vi "Preference_Panel.vi"(0 "Mode":T3) -> ()   [LabVIEW 2015]
uses:
  Anemometry Sub Vis/Controls/Server_Comms.ctl
  Anemometry Sub Vis/Controls/Preference_Mode.ctl
  Anemometry Sub Vis/Controls/EnFlo_Data_Folder_Setup.ctl
  Camera Server/sub vis/List of Cameras.ctl
  Anemometry Sub Vis/File/Setup_Filetype.ctl
  Anemometry Sub Vis/Controls/Overhead.ctl
  ADAM Client/Sub VIs/ADAM Controls/Ch_description_ADAM.ctl
  ADAM Client/Sub VIs/ADAM Controls/Module_type_ADAM.ctl
  ADAM Client/Sub VIs/ADAM Controls/Function_ADAM.ctl
  ADAM Client/Sub VIs/ADAM Controls/Channel_State.ctl
  ADAM Client/Sub VIs/ADAM Controls/Calib_type_ADAM.ctl
  ADAM Client/Sub VIs/ADAM Controls/Address.ctl
  Anemometry Sub Vis/Globals/Constants_global.vi
  Anemometry Sub Vis/Globals/Preference_global.vi
  Anemometry Sub Vis/Globals/Trav_pos_global.vi
  Camera Server/Globals/CamServer global.vi
  Anemometry Sub Vis/Acquisition/PWA/PWAtasksGLOBAL.vi
panel:
  in  "Cameras to Log":T1[](array[typedef])
  out "Preferences for computer":string
  in  "Log Cameras if available":bool
  in  "Use New Collision Code":bool
  in  "Traverse to Traverse Collision Detection":bool
  in  "DataTranslation Device No.":u32=20
  in  "Reset Email Counter":bool
  in  "EnFlo_Data_Folder_Setup":T2="EnFlo_Data on Server"
  in  "Post Processing Machine":bool
  in  "Analogue Device Serial No.":string="1188AB4"
  in  "PWA Device Serial No.":string="1187C98"
  in  "ADAM Setup File":u16(ring) items=["Scani_Valve.xls", "Current_Setup.xls"]
  in  "Default Source Establishment Time (s)":dbl=20.0
  out "This Machine's IP Number":string
  in  "Rig Setup":u16(ring) items=["3_x_2_tunnel", "A_Tunnel", "Adam_Sayer_Desk", "ADAM_Server", "Aero_Tunnel", "Alex_Desktop", "B_Tunnel", "Calibration_Tunnel", "Contact_Conductance", "D_Tunnel", "EnFlo_Tunnel", "Frauke_Desktop", "Fruit_Rig", "iMac_G5_2", "iMacDuo1", "Matteo's_desktop", "Matteo_PC", "Nick_PC-2", "Paul_Desk-Paul_Desk_Machine", "Paul_Hayden-Desk", "Paul_N_Desk_Machine_2", "phtest", "Post_Processing_Machine", "PowerBook_G4_1", "PowerBook_G4_2", "Syn_jet_rig", "Tank", "tdf", "Tom_Desk", "Towing_tank", "--New Rig Setup--"]
  in  "Default Traverse Name":u16(ring) items=["A_Tunnel", "Aero_Laser", "Aero_ThroughWall", "Aero_Tunnel", "Angle_Calibrator", "B_Tunnel", "D_Tunnel", "Dummy_Traverse", "EnFlo_Stack", "EnFlo_Tunnel", "EnFlo_Turntable", "Laser_Meas_Traverse", "mohd_setup", "Paul_Desk_Test", "PIV_Traverse", "--New Traverse Setup--"]
  in  "OK":bool
  in  "% Error From First Calib":dbl=10.0 format="%.1f"
  in  "% Error From Previous Calib":dbl=0.5 format="%.1f"
  out "Templates":path=path "/G4_2_HD/Applications (Mac OS 9)/EnFlo Software/Anemometry/Anemometry Sub Vis/Templates"
  in  "Data Folder":path
  out "EnFlo SW Preferences":path=path "/G4_2_HD/Applications (Mac OS 9)/LabVIEW 5.1/EnFlo SW Preferences"
  in  "Tunnel Speed Control":bool
  in  "SMTP server IP address":string
  in  "Abs Press (mbar)":string="Froude:NPL:Atmos_Press"
  in  "Temperature":string="EnFlo Tun:Inlet Heater:Av Temp"
  in  "Server port number":u32=3363
  in  "Server address":string
  in  "LabVIEW Administrators":string[](array[string])=["", "", "", "", "", "", "", "", "", "", "", "", "", "", "", "", "", "", "", ""]
  in  "Server Comms":T4=enum."Do Not Link To Server"
  # "Server Computer Peferences"
  # "Multi Run Preferences"
  # "Warning Levels for Autocalibration Changes"
  # "Email Peferences"
  # "Deg C"
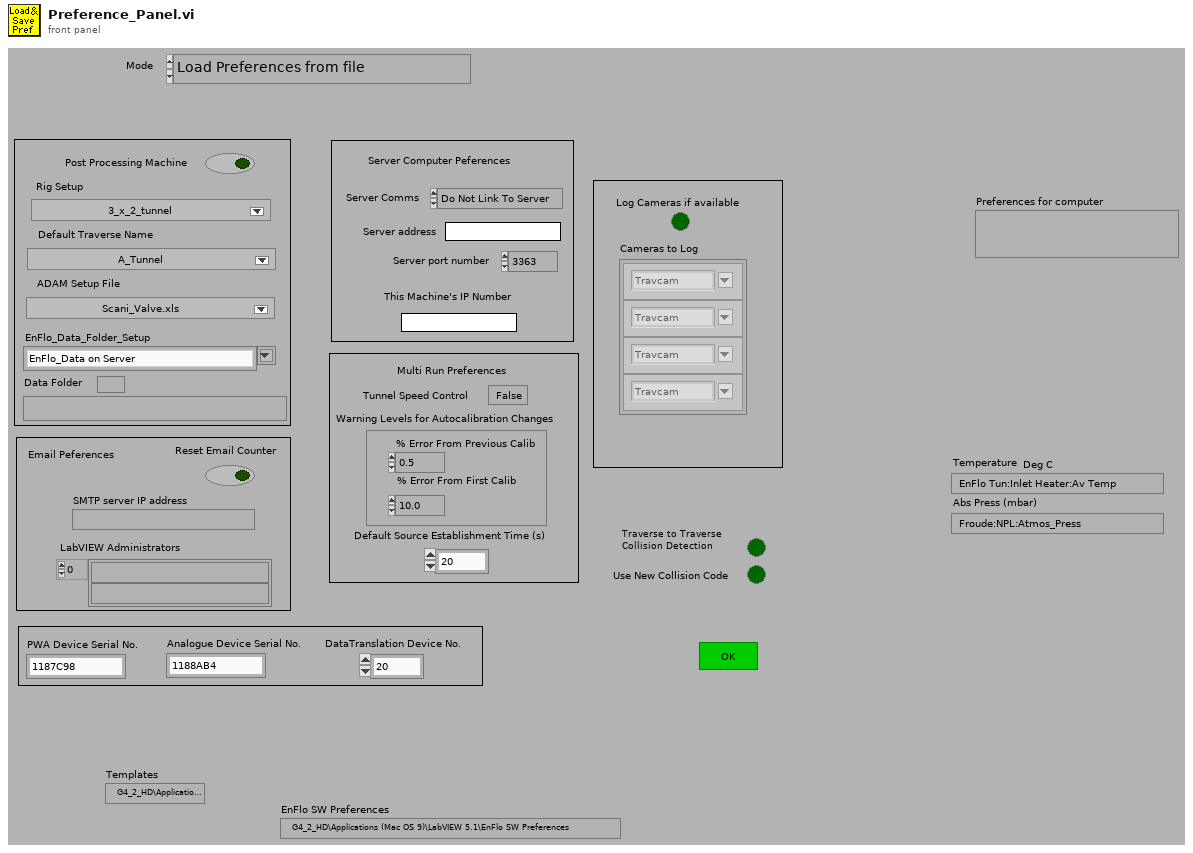
[diagram p1: front panel]
types:
  T1 = typedef "List of Cameras.ctl" = string
  T2 = typedef "EnFlo_Data_Folder_Setup.ctl" = string
  T3 = typedef "Preference_Mode.ctl" = enum16{"Load Preferences from file", "Save Preferences to file", "Load, Edit then Save"}
  T4 = typedef "Server_Comms.ctl" = enum16{"Server Link Healthy", "Do Not Link To Server"}
  T5 = enum16{"Zero or one", "One", "Zero or more", "One or more"}
  T6 = enum8{"Enabled", "Disabled", "Disabled and Grayed Out"}
  T7 = typedef "Setup_Filetype.ctl" = enum16{"Measurement Setups", "Calibration Setups", "General", "Results File Plotter Setups", "Speed Calib Tweaks"}
  T8 = typedef "Overhead.ctl" = enum16{"Update total times", "Read Current Overhead", "Re Scale totals to 3 hrs", "Initialise totals to 3hr"}
  T9 = typedef "Calib_type_ADAM.ctl" = enum16{"Raw", "Bx + A", "Cx^2 + Bx + A", "Dx^3 + Cx^2 + Bx + A", "In Band", "Hi-Tec Q", "Hi-Tec M_dot", "Text"}
  T10 = typedef "Module_type_ADAM.ctl" = string
  T11 = typedef "Channel_State.ctl" = enum16{"On", "Off", "Always On", "Always Off"}
  T12 = typedef "LVDateTimeRec.ctl" = cluster{"fractional second":dbl, "second":i32, "minute":i32, "hour":i32, "day of month":i32, "month":i32, "year":i32, "day of week":i32, "day of year":i32, "DST":i32}
  T13 = typedef "Ch_description_ADAM.ctl" = cluster{"Ch Name":string, "Type":T10, "Function":T14, "Ch State":T11, "Calibration type":T9, "A":dbl, "B":dbl, "C":dbl, "D":dbl, "Comments":string, "Address":T15, "String":string, "Duty":u16}
  T14 = typedef "Function_ADAM.ctl" = enum16{"Analogue Input", "Digital Input", "Event counter", "Event rate", "Analogue Output", "Digital Output", "Relay Output"}
  T15 = typedef "Address.ctl" = cluster{"Main":i32, "Ch.":i32, "Sub":i32, "Port Name":string}
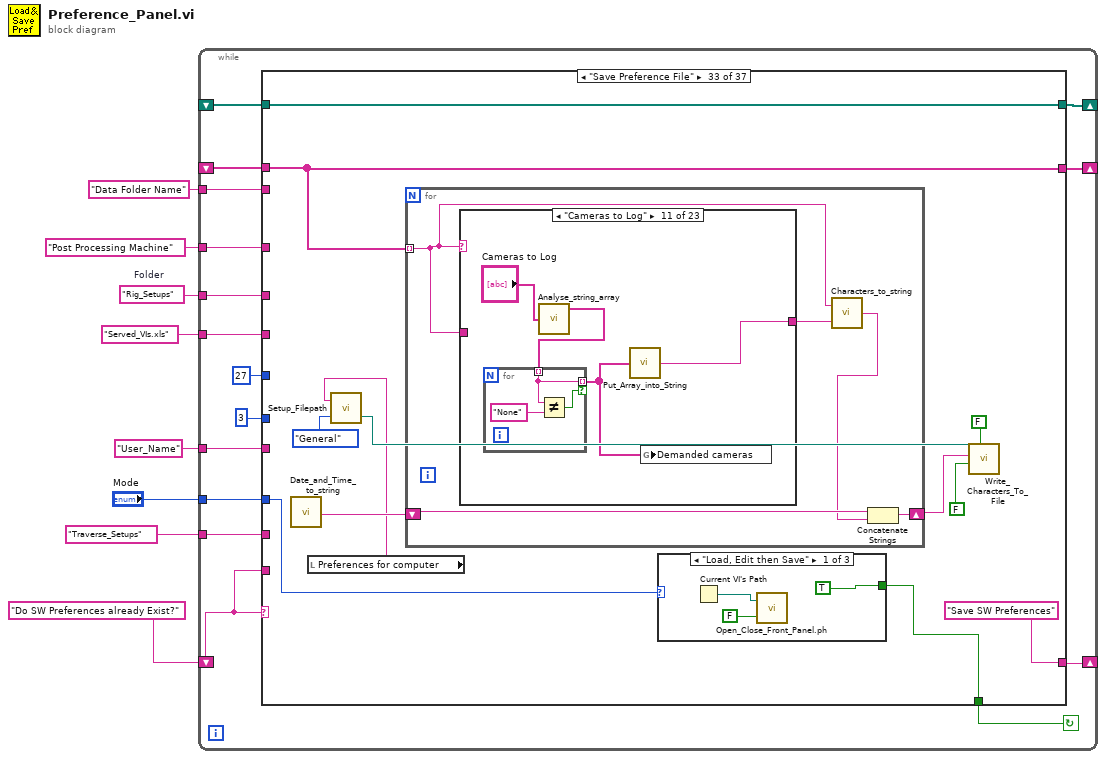
[diagram p0: block diagram]
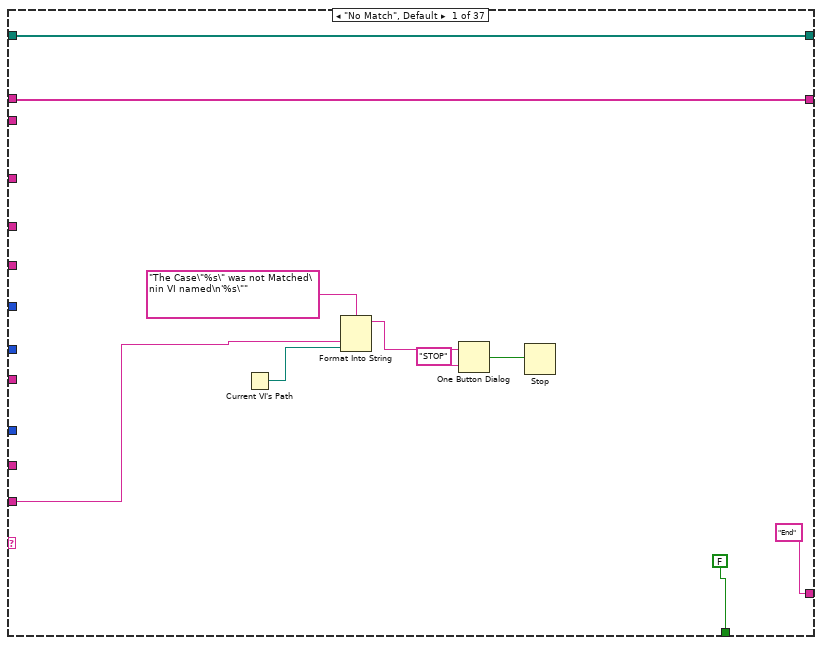
[diagram p2: hidden frame]
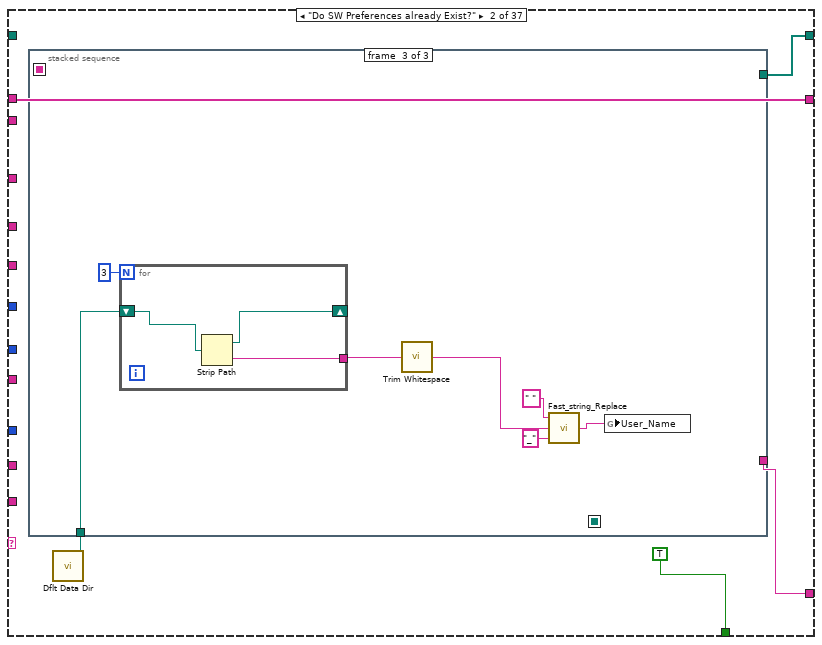
[diagram p3: hidden frame]
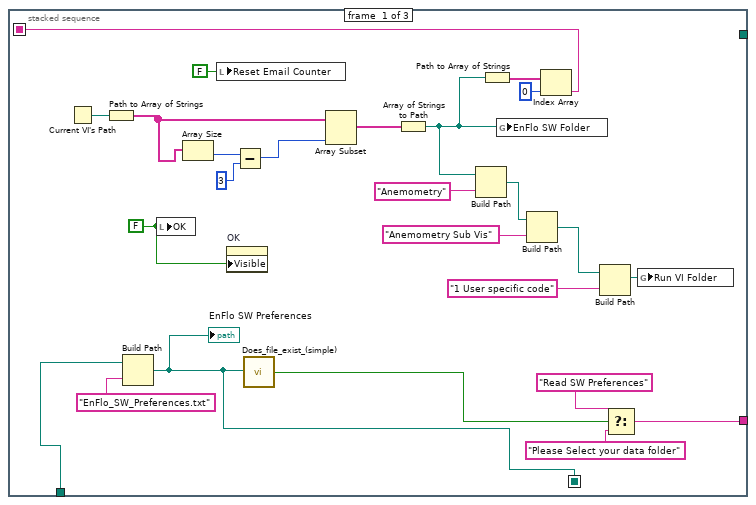
[diagram p4: hidden frame]
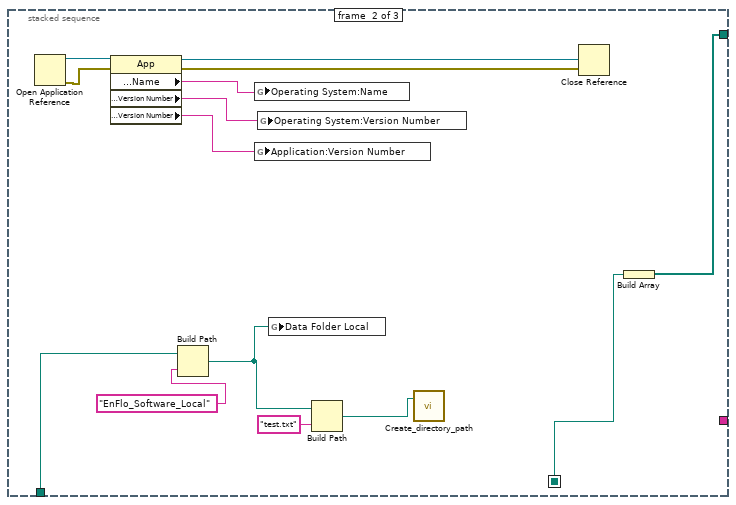
[diagram p5: hidden frame]
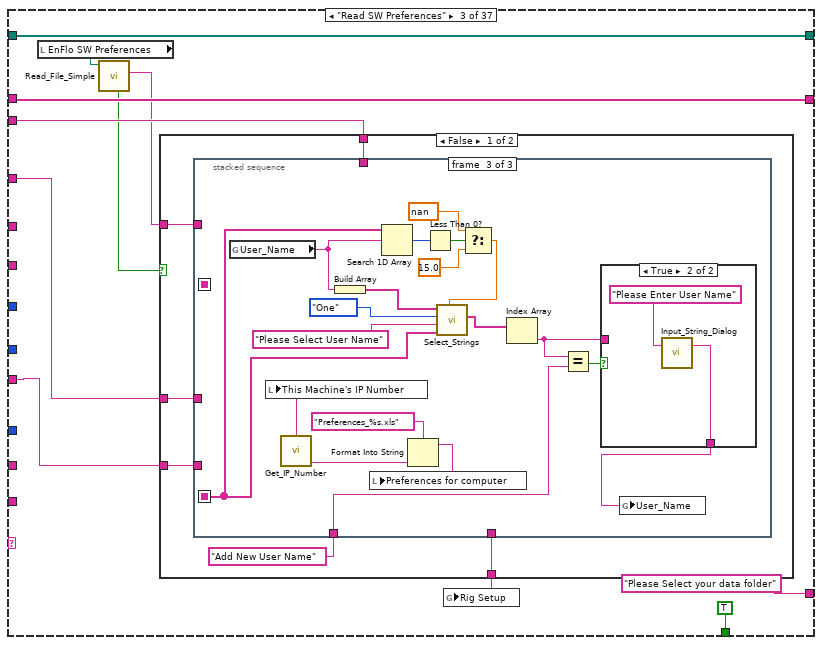
[diagram p6: hidden frame]
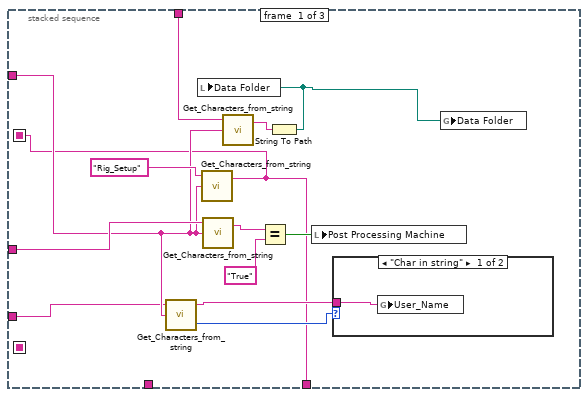
[diagram p7: hidden frame]
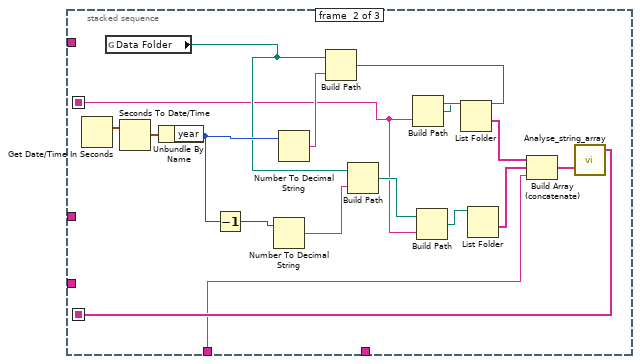
[diagram p9: hidden frame]
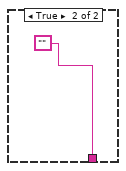
[diagram p11: hidden frame]
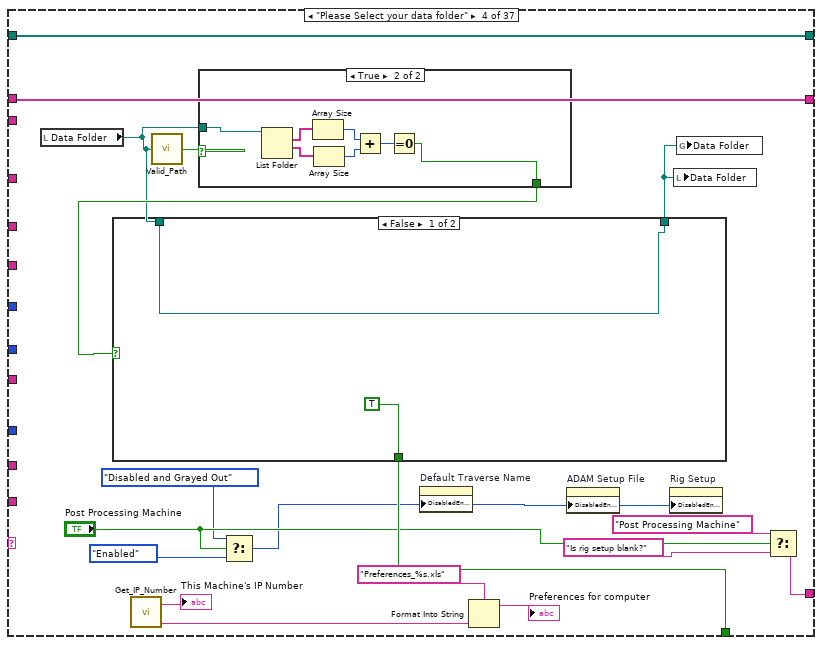
[diagram p12: hidden frame]
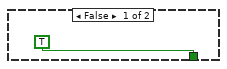
[diagram p13: hidden frame]
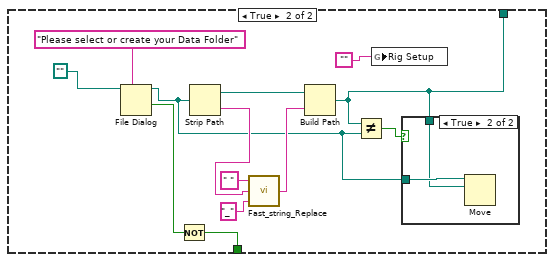
[diagram p14: hidden frame]
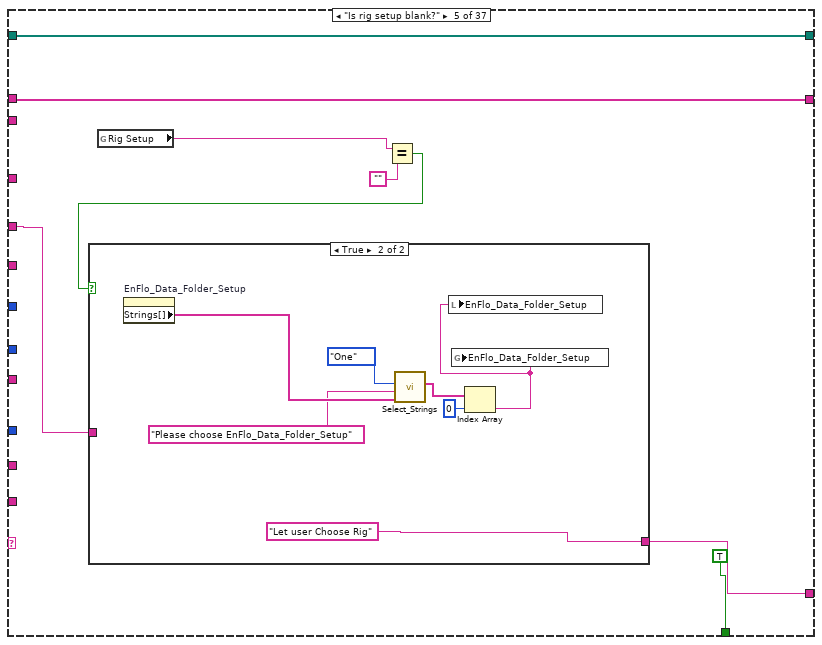
[diagram p16: hidden frame]
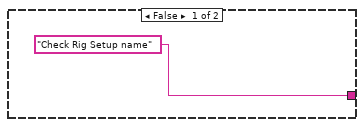
[diagram p17: hidden frame]
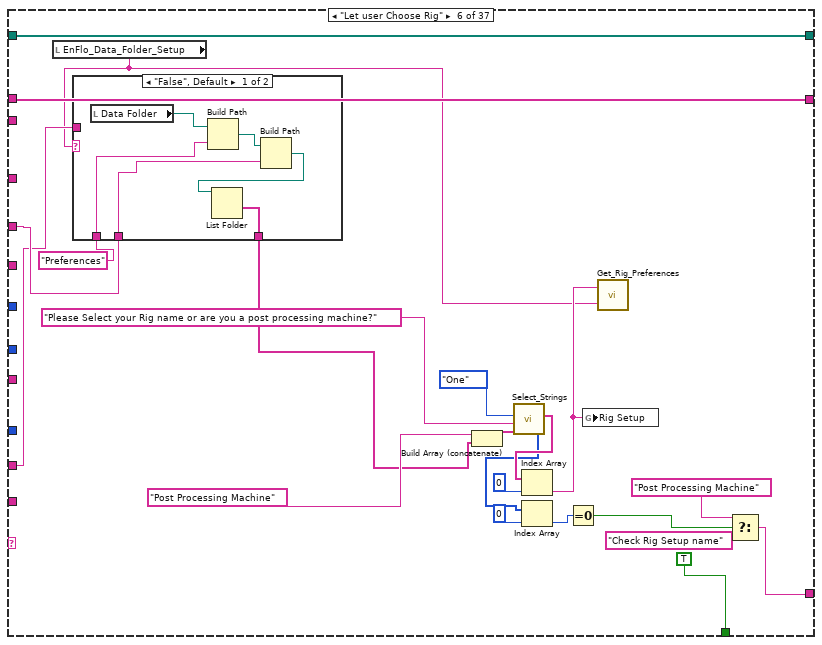
[diagram p18: hidden frame]
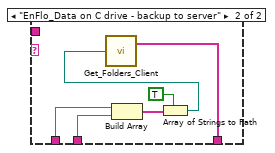
[diagram p19: hidden frame]
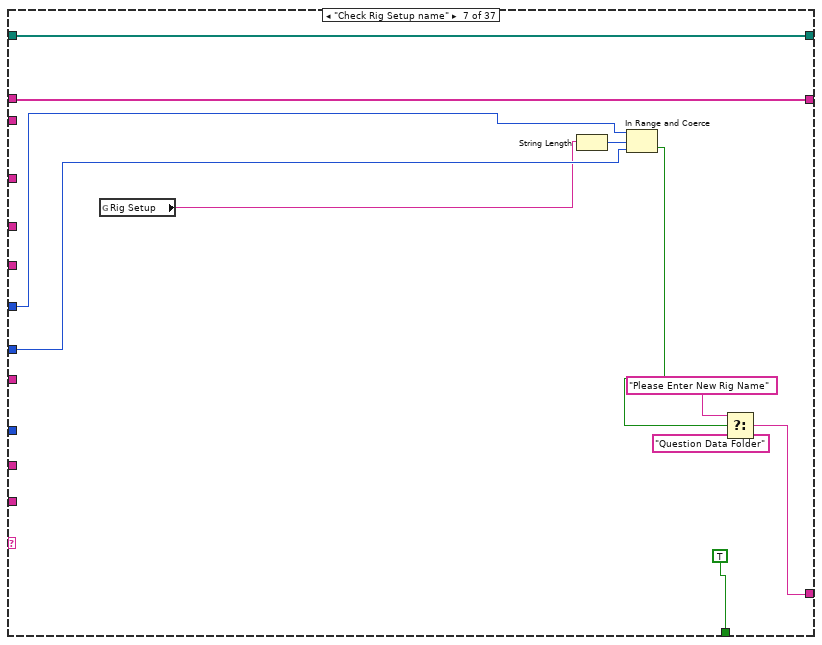
[diagram p20: hidden frame]
diagram:
  w4 = "Rig_Setups"  # Folder
  n1 = while {
    shift-left: _ -> [w21]
    shift-right: [w22] -> _
    shift-left: "Do SW Preferences already Exist?" -> [w10]
    shift-right: [w23] -> _
    tunnel: "Mode" -> [w20]
    tunnel: "Data Folder Name" ("Label for characters") -> [w19]
    tunnel: "Served_VIs.xls" ("Substring") -> [w18]
    tunnel: w4 -> [w15]
    tunnel: "Traverse_Setups" ("name or relative path") -> [w14]
    shift-right: [w13] -> _
    shift-left: _ -> [w12]
    tunnel: "Post Processing Machine" ("Label for characters") -> [w11]
    tunnel: "User_Name" ("Label for characters") -> [w9]
    stop <- w24 continue-if-true
    n2 = case shown="\"Save Preference File\"" w10 {
      tunnel: [FALSE TRUE TRUE w171 TRUE TRUE TRUE TRUE TRUE TRUE TRUE TRUE TRUE TRUE TRUE TRUE TRUE TRUE TRUE TRUE TRUE TRUE TRUE TRUE TRUE TRUE TRUE TRUE TRUE TRUE TRUE TRUE w938 TRUE TRUE TRUE FALSE] -> w24
      tunnel: ["End" w37 "Please Select your data folder" w168 w203 w236 w253 w264 w283 "Update Constants Global" ("f") "Copy Preferences?" "Copy Preferences?" w414 w431 "Install Preference files" "Install Adam table files" "Install Adam setup files" "Choose ADAM Setup file" "Preference files continued" "Variable Names" w611 w631 "Please Enter new  Traverse Setup" w718 "Create Traverse setup" ("f") "Check file permission status" w815 w846 w866 w886 w902 "Save Preference File" "Save SW Preferences" w1028 w1042 "Initialise Globals" "End"] -> w23
      tunnel: [w26 w38 w98 w177 w209 w239 w262 w272 w285 w350 w378 w401 w412 w435 w493 w508 w533 w552 w574 w584 w616 w638 w706 w720 w754 w771 w816 w851 w871 w894 w907 w927 w944 w1036 w1043 w1095 w1153] -> w22
      tunnel: w21 -> [w26 w38 w98 w177 w209 w239 w262 w272 w285 w350 w378 w401 w412 w435 w493 w508 w533 w552 w574 w584 _ w638 w706 w720 w754 w771 w816 w851 w871 w894 w907 w927 w944 w1036 w1043 w1095 w1153]
      tunnel: w10 -> [w29 _ _ _ _ _ _ _ _ _ _ _ _ _ _ _ _ _ _ _ _ _ _ _ _ _ _ _ _ _ _ _ _ _ _ _ _]
      tunnel: w20 -> [_ _ _ _ _ _ _ _ _ _ _ _ _ _ _ _ _ _ _ _ w610 _ _ _ _ _ w814 _ _ _ _ _ w939 _ _ _ _]
      tunnel: w19 -> [_ _ w95 _ _ _ _ _ _ _ _ _ _ _ _ _ _ _ _ _ _ _ _ _ _ _ _ _ _ _ _ _ _ w1027 _ _ _]
      tunnel: w18 -> [_ _ _ _ _ _ _ _ _ _ _ _ _ _ _ w503 _ _ _ _ _ _ _ _ _ _ _ _ _ _ _ _ _ _ _ w1087 _]
      tunnel: 3 ("lower limit") -> [_ _ _ _ _ _ w258 _ w282 _ _ _ _ _ _ _ _ _ _ _ _ _ _ w717 _ _ _ _ _ _ _ _ _ _ _ _ _]
      tunnel: 27 ("upper limit") -> [_ _ _ _ _ _ w259 _ w281 _ _ _ _ _ _ _ _ _ _ _ _ _ _ w716 _ _ _ _ _ _ _ _ _ _ _ _ _]
      tunnel: w15 -> [_ _ _ _ w206 w224 _ _ _ w338 w366 _ _ w434 _ _ _ _ _ _ _ _ _ _ _ _ _ _ _ _ _ _ _ _ _ _ _]
      tunnel: w14 -> [_ _ _ _ _ w221 _ _ _ _ _ _ _ _ _ _ _ _ _ _ _ _ w704 _ w741 _ _ _ _ _ _ _ _ _ _ _ _]
      tunnel: [w25 w35 w94 w172 w204 w238 w261 w271 w277 w336 w363 w390 w413 w436 w486 w500 w526 w549 w560 w576 w603 w634 w703 w712 w740 w767 path[] [] w843 w863 w889 w905 w926 w937 w1024 w1041 w1089 w1151] -> w13
      tunnel: w12 -> [w25 _ w94 w172 w204 w238 w261 w271 w277 w336 w363 w390 w413 w436 w485 w502 w526 w550 w560 w578 w603 w635 w703 w712 w740 w768 w813 w843 w863 w889 w905 w926 w937 w1024 w1041 w1089 w1151]
      tunnel: w11 -> [_ _ w93 _ _ _ _ _ _ _ _ _ _ _ _ _ _ _ _ _ _ _ _ _ _ _ _ _ _ _ _ _ _ w1018 _ _ _]
      tunnel: w9 -> [_ _ w89 _ _ _ _ _ _ _ _ _ _ _ _ _ _ _ _ _ _ _ _ _ _ _ _ _ _ _ _ _ _ w1017 _ _ _]
      frame "No Match", Default {
        n3 = Current VI's Path() -> (path=w34:path)
        n4 = Format Into String(format string="The Case\"%s\" was not Matched\nin VI named\n'%s\"" ("Format String"), w29, w34) -> (resulting string=w31:string)  [unwired: 2 in, 1 out]
        n5 = One Button Dialog(message=w31, button name ("OK")="STOP") -> (true=w33:bool)
        n6 = Stop(stop? (T)=w33) -> ()
      }
      frame "Do SW Preferences already Exist?" {
        n7 = call <vilib>:"Dflt Data Dir.vi"() -> ("App:Default Data Directory"=w36:path)
        n8 = stacked-sequence {
          seq-local: [w44 _ _] -> [_ _ _]
          seq-local: [w42 _ _] -> [_ w70 _]
          tunnel: [w48 _ _] -> w37
          tunnel: w36 -> [w43 w68 w84]
          tunnel: [_ w71 _] -> w35
          frame #0 {
            w41 = FALSE ("OK")
            n9 = Current VI's Path() -> (path=w62:path)
            n10 = Path to Array of Strings(0:w62) -> (2:w59:string[])  [unwired: 1 out]
            n11 = Build Path(base path=w43, name or relative path="EnFlo_SW_Preferences.txt") -> (appended path=w42:path)
            "EnFlo SW Preferences" <- w42
            n12 = local write "OK"(w41) -> ()
            n13 = Array Size(array=w59) -> (size(s)=w61:i32)
            n14 = local write "Reset Email Counter"(FALSE ("Reset Email Counter")) -> ()
            n15 = property on="OK" class="Bool (strict)"("Visible"=w41) -> ()  [unwired: 2 in, 2 out]
            n16 = Subtract(x=w61, y=3) -> (x-y=w57:i32)
            n17 = call "Does_file_exist_(simple).vi"("Pathname"=w42) -> ("exists?"=w63:bool)
            n18 = Array Subset(array=w59, length=w57) -> (w58:string[])  [unwired: 1 in]
            n19 = Array of Strings to Path(0:w58) -> (2:w45:path)  [unwired: 1 out]
            n20 = Build Path(base path=w45, name or relative path="Anemometry") -> (appended path=w54:path)
            n21 = Path to Array of Strings(0:w45) -> (2:w46:string[])  [unwired: 1 out]
            n22 = global write "Constants_global.vi" "EnFlo SW Folder"(w45) -> ()
            n23 = Build Path(base path=w54, name or relative path="Anemometry Sub Vis") -> (appended path=w52:path)
            n24 = Index Array(array=w46, index=0) -> (element=w44:string)
            n25 = Build Path(base path=w52, name or relative path="1 User specific code") -> (appended path=w51:path)
            n26 = Select(t="Read SW Preferences", s=w63, f="Please Select your data folder") -> (s? t:f=w48:string)
            n27 = global write "Constants_global.vi" "Run VI Folder"(w51) -> ()
          }
          frame #1 {
            n28 = Open Application Reference() -> (0:w75:errorcluster, 3:w78:refnum<vi>)  [unwired: 1 in, 3 out]
            n29 = property class="App"(reference=w78, error in=w75) -> (reference out=w77:refnum<vi>, error out=w76:errorcluster, "Operating System:Name"=w72:string, "Operating System:Version Number"=w74:string, "Application:Version Number"=w73:string)
            n30 = Build Path(base path=w68, name or relative path="EnFlo_Software_Local" ("element")) -> (appended path=w67:path)
            n31 = global write "Preference_global.vi" "Operating System:Name"(w72) -> ()
            n32 = global write "Preference_global.vi" "Application:Version Number"(w73) -> ()
            n33 = global write "Preference_global.vi" "Operating System:Version Number"(w74) -> ()
            n34 = global write "Constants_global.vi" "Data Folder Local"(w67) -> ()
            n35 = Build Path(base path=w67, name or relative path="test.txt") -> (appended path=w65:path)
            n36 = call "Create_directory_path.vi"("Path name"=w65) -> ()  [unwired: 1 in, 2 out]
            n37 = Close Reference(reference=w77, error in (no error)=w76) -> ()  [unwired: 1 out]
            n38 = Build Array(w70) -> (w71:path[])
          }
          frame #2 {
            n39 = for {
              N: 3 -> [_]
              shift-right: [w88] -> _
              shift-left: w84 -> [w87]
              tunnel: [w86] -> w80
              n40 = Strip Path(path=w87) -> (stripped path=w88:path, name=w86:string)
            }
            n41 = call <vilib>:"Trim Whitespace.vi"("string"=w80) -> ("trimmed string"=w79:string)  [unwired: 1 in]
            n42 = call "Fast_string_Replace.vi"("Replace match with:"="_", "Input String"=w79, "regular expression"=" ") -> ("Output String"=w81:string)  [unwired: 1 in, 1 out]
            n43 = global write "Preference_global.vi" "User_Name"(w81) -> ()
          }
        }
      }
      frame "Read SW Preferences" {
        n44 = local read "EnFlo SW Preferences"() -> (w97:path)
        n45 = call "Read_File_Simple.vi"("Filename"=w97) -> ("Error?"=w91:bool, "string"=w92:string)  [unwired: 2 in, 6 out]
        n46 = case shown="False" w91 {
          tunnel: w95 -> [w105 _]
          tunnel: w93 -> [w104 _]
          tunnel: w92 -> [w102 _]
          tunnel: [w103 ""] -> w90
          tunnel: w89 -> [w101 _]
          frame False {
            n47 = stacked-sequence {
              seq-local: [w106 _ _] -> [_ w126 _]
              seq-local: [_ w121 _] -> [_ _ w146]
              tunnel: w105 -> [w117 _ _]
              tunnel: w104 -> [w114 _ _]
              tunnel: [w106 _ _] -> w103
              tunnel: w102 -> [w110 _ _]
              tunnel: w101 -> [w109 _ _]
              tunnel: "Add New User Name" -> [_ w120 w151]
              frame #0 {
                n48 = call "Get_Characters_from_string.vi"("Input string"=w110, "Variable name"=w109) -> ("Status"=w108:enum16{"Char in string", "Char not in string"}, "Value"=w107:string)  [unwired: 1 in]
                n49 = call "Get_Characters_from_string.vi"("Input string"=w110, "Variable name"="Rig_Setup" ("Label for characters")) -> ("Value"=w106:string)  [unwired: 1 in, 1 out]
                n50 = call "Get_Characters_from_string.vi"("Input string"=w110, "Variable name"=w114) -> ("Value"=w113:string)  [unwired: 1 in, 1 out]
                n51 = call "Get_Characters_from_string.vi"("Input string"=w110, "Variable name"=w117) -> ("Value"=w118:string)  [unwired: 1 in, 1 out]
                n52 = Equal?(x=w113, y="True") -> (x = y?=w111:bool)
                n53 = String To Path(string=w118) -> (path=w116:path)
                n54 = local write "Data Folder"(w116) -> ()
                n55 = local write "Post Processing Machine"(w111) -> ()
                n56 = case shown="\"Char in string\"" w108 {
                  tunnel: w107 -> [w119 _]
                  frame "Char in string" {
                    n57 = global write "Preference_global.vi" "User_Name"(w119) -> ()
                  }
                  frame "Char not in string" {
                  }
                }
                n58 = global write "Constants_global.vi" "Data Folder"(w116) -> ()
              }
              frame #1 {
                n59 = Get Date/Time In Seconds() -> (seconds since 1Jan1904=w136:timestamp)
                n60 = global read "Constants_global.vi" "Data Folder"() -> (w129:path)
                n61 = Seconds To Date/Time(time stamp (now)=w136) -> (date time rec=w135:T12)  [unwired: 1 in]
                n62 = Unbundle By Name(w135) -> ("year"=w134:i32)
                n63 = Decrement(x=w134) -> (x-1=w133:i32)
                n64 = Number To Decimal String(number=w133) -> (decimal integer string=w128:string)  [unwired: 1 in]
                n65 = Number To Decimal String(number=w134) -> (decimal integer string=w132:string)  [unwired: 1 in]
                n66 = Build Path(base path=w129, name or relative path=w132) -> (appended path=w131:path)
                n67 = Build Path(base path=w129, name or relative path=w128) -> (appended path=w127:path)
                n68 = Build Path(base path=w131, name or relative path=w126) -> (appended path=w130:path)
                n69 = Build Path(base path=w127, name or relative path=w126) -> (appended path=w125:path)
                n70 = List Folder(path=w130) -> (folder names=w124:string[])  [unwired: 3 in, 3 out]
                n71 = List Folder(path=w125) -> (folder names=w123:string[])  [unwired: 3 in, 3 out]
                n72 = Build Array (concatenate)(w124, w123, w120) -> (w122:string[])
                n73 = call "Analyse_string_array.vi"("String array"=w122) -> ("Unique strings"=w121:string[])  [unwired: 1 in, 1 out]
              }
              frame #2 {
                n74 = global read "Preference_global.vi" "User_Name"() -> (w147:string)
                n75 = call "Get_IP_Number.vi"() -> ("Computer Name"=w139:string, "IP Number"=w140:string)
                n76 = local write "This Machine's IP Number"(w140) -> ()
                n77 = Build Array(w147) -> (w154:string[])
                n78 = Search 1D Array(1D array=w146, element=w147) -> (index of element=w145:i32)  [unwired: 1 in]
                n79 = Format Into String(format string="Preferences_%s.xls" ("name or relative path"), w139) -> (resulting string=w138:string)  [unwired: 2 in, 1 out]
                n80 = local write "Preferences for computer"(w138) -> ()
                n81 = Less Than 0?(x=w145) -> (x < 0?=w144:bool)
                n82 = Select(t=nan ("Timeout (s)"), s=w144, f=15.0 ("Timeout (s)")) -> (s? t:f=w141:dbl)
                n83 = call "Select_Strings.vi"("Timeout (s)"=w141, "Available Ch names"=w146, "Message"="Please Select User Name", "Selector mode"=T5."One", "Desired Ch names (in)"=w154) -> ("Selected Channel Names"=w152:string[])  [unwired: 1 in, 2 out]
                n84 = Index Array(array=w152) -> (element=w148:string)  [unwired: 1 in]
                n85 = Equal?(x=w148, y=w151) -> (x = y?=w150:bool)
                n86 = case shown="True" w150 {
                  tunnel: [w156 w157] -> w149
                  tunnel: w148 -> [w156 _]
                  frame False {
                  }
                  frame True {
                    n87 = call "Input_String_Dialog.vi"("Message to user"="Please Enter User Name") -> ("Output string"=w157:string)  [unwired: 1 in, 1 out]
                  }
                }
                n88 = global write "Preference_global.vi" "User_Name"(w149) -> ()
              }
            }
          }
          frame True {
          }
        }
        n89 = global write "Preference_global.vi" "Rig Setup"(w90) -> ()
      }
      frame "Please Select your data folder" {
        n90 = local read "Data Folder"() -> (w173:path)
        n91 = call "Get_IP_Number.vi"() -> ("Computer Name"=w162:string, "IP Number"=→"This Machine's IP Number":string)
        n92 = call "Valid_Path.vi"("Filename"=w173) -> ("Valid Path?"=w175:bool)
        n93 = case shown="True" w175 {
          tunnel: [TRUE ("status") w179] -> w174
          tunnel: w173 -> [_ w185]
          frame False {
          }
          frame True {
            n94 = List Folder(path=w185) -> (filenames=w183:string[], folder names=w184:string[])  [unwired: 1 in, 4 out]
            n95 = Array Size(array=w183) -> (size(s)=w181:i32)
            n96 = Array Size(array=w184) -> (size(s)=w182:i32)
            n97 = Add(x=w181, y=w182) -> (x+y=w180:i32)
            n98 = Equal To 0?(x=w180) -> (x = 0?=w179:bool)
          }
        }
        n99 = case shown="False" w174 {
          tunnel: [w187 w191] -> w176
          tunnel: w173 -> [w187 _]
          tunnel: [TRUE w189] -> w171
          frame False {
          }
          frame True {
            n100 = File Dialog(7:"Please select or create your Data Folder" ("prompt"), 11:path "") -> (1:w190:bool, 3:w192:path)  [unwired: 1 in, 6 out]
            n101 = Not(x=w190) -> (.not. x?=w189:bool)
            n102 = Strip Path(path=w192) -> (stripped path=w196:path, name=w195:string)
            n103 = call "Fast_string_Replace.vi"("Replace match with:"="_", "Input String"=w195, "regular expression"=" ") -> ("Output String"=w194:string)  [unwired: 2 out]
            n104 = Build Path(base path=w196, name or relative path=w194) -> (appended path=w191:path)
            n105 = Not Equal?(x=w191, y=w192) -> (x != y?=w193:bool)
            n106 = global write "Preference_global.vi" "Rig Setup"("") -> ()
            n107 = case shown="True" w193 {
              tunnel: w192 -> [_ w202]
              tunnel: w191 -> [_ w201]
              frame False {
              }
              frame True {
                n108 = Move(source path=w202, 10:w201) -> ()  [unwired: 1 in, 5 out]
              }
            }
          }
        }
        n109 = Select(t=T6."Disabled and Grayed Out" ("Disabled"), s="Post Processing Machine", f=T6."Enabled" ("Disabled")) -> (s? t:f=w164:T6)
        n110 = property on="Default Traverse Name" class="Ring (strict)"("DisabledEnum"=w164) -> ()  [unwired: 2 in, 2 out]
        n111 = Format Into String(format string="Preferences_%s.xls" ("name or relative path"), w162) -> (resulting string=→"Preferences for computer":string)  [unwired: 2 in, 1 out]
        n112 = property on="ADAM Setup File" class="Ring (strict)"("DisabledEnum"=w164) -> ()  [unwired: 2 in, 2 out]
        n113 = property on="Rig Setup" class="Ring (strict)"("DisabledEnum"=w164) -> ()  [unwired: 2 in, 2 out]
        n114 = local write "Data Folder"(w176) -> ()
        n115 = global write "Constants_global.vi" "Data Folder"(w176) -> ()
        n116 = Select(t="Post Processing Machine", s="Post Processing Machine", f="Is rig setup blank?") -> (s? t:f=w168:string)
      }
      frame "Is rig setup blank?" {
        n117 = global read "Preference_global.vi" "Rig Setup"() -> (w205:string)
        n118 = Equal?(x=w205, y="") -> (x = y?=w207:bool)
        n119 = case shown="True" w207 {
          tunnel: w206 -> [_ _]
          tunnel: ["Check Rig Setup name" ("t") "Let user Choose Rig"] -> w203
          frame False {
          }
          frame True {
            n120 = property on="EnFlo_Data_Folder_Setup" class="CmbBox (strict)"() -> ("Strings[]"=w216:string[])  [unwired: 2 in, 2 out]
            n121 = call "Select_Strings.vi"("Available Ch names"=w216, "Message"="Please choose EnFlo_Data_Folder_Setup", "Selector mode"=T5."One") -> ("Selected Channel Names"=w214:string[])  [unwired: 3 in, 2 out]
            n122 = Index Array(array=w214, index=0) -> (element=w212:string)
            n123 = local write "EnFlo_Data_Folder_Setup"(w212) -> ()
            n124 = global write "Preference_global.vi" "EnFlo_Data_Folder_Setup"(w212) -> ()
          }
        }
      }
      frame "Let user Choose Rig" {
        n125 = local read "EnFlo_Data_Folder_Setup"() -> (w219:T2)
        n126 = case shown="\"False\", Default" w219 {
          tunnel: "Preferences" ("name or relative path") -> [w244 w247]
          tunnel: w224 -> [w243 w252]
          tunnel: [w242 w249] -> w222
          tunnel: w221 -> [_ _]
          frame "False", Default {
            n127 = local read "Data Folder"() -> (w245:path)
            n128 = Build Path(base path=w245, name or relative path=w244) -> (appended path=w246:path)
            n129 = Build Path(base path=w246, name or relative path=w243) -> (appended path=w241:path)
            n130 = List Folder(path=w241) -> (folder names=w242:string[])  [unwired: 1 in, 5 out]
          }
          frame "EnFlo_Data on C drive - backup to server" {
            n131 = Build Array(w247, w252) -> (w251:string[])
            n132 = Array of Strings to Path(0:w251, 1:TRUE ("relative")) -> (2:w248:path)
            n133 = call "Get_Folders_Client.vi"("Relative Path"=w248) -> ("Folder Names"=w249:string[])  [unwired: 1 out]
          }
        }
        n134 = Build Array (concatenate)("Post Processing Machine", w222) -> (w229:string[])
        n135 = call "Select_Strings.vi"("Available Ch names"=w229, "Message"="Please Select your Rig name or are you a post processing machine?", "Selector mode"=T5."One") -> ("Ch Indicies Choosen"=w226:i32[], "Selected Channel Names"=w228:string[])  [unwired: 3 in, 1 out]
        n136 = Index Array(array=w228, index=0) -> (element=w220:string)
        n137 = Index Array(array=w226, index=0) -> (element=w225:i32)
        n138 = Equal To 0?(x=w225) -> (x = 0?=w235:bool)
        n139 = global write "Preference_global.vi" "Rig Setup"(w220) -> ()
        n140 = call "Get_Rig_Preferences.vi"("EnFlo_Data_Folder_Setup"=w219, "Rig Setup"=w220) -> ()  [unwired: 1 in]
        n141 = Select(t="Post Processing Machine", s=w235, f="Check Rig Setup name") -> (s? t:f=w236:string)
      }
      frame "Check Rig Setup name" {
        n142 = global read "Preference_global.vi" "Rig Setup"() -> (w254:string)
        n143 = String Length(string=w254) -> (length=w260:i32)
        n144 = In Range and Coerce(upper limit=w259, x=w260, lower limit=w258) -> (In Range?=w257:bool)  [unwired: 1 out]
        n145 = Select(t="Please Enter New Rig Name", s=w257, f="Question Data Folder") -> (s? t:f=w253:string)
      }
      frame "Question Data Folder" {
        (unwired) "Question Data Folder"
        n146 = local read "Data Folder"() -> (w270:path)
        n147 = Format Into String(format string="Is the Data Folder\n%s\nCorrect?" ("message"), w270) -> (resulting string=w268:string)  [unwired: 2 in, 1 out]
        n148 = Two Button Dialog(message=w268, 1:"No, let me change it" ("F button name (\"Cancel\")"), 2:"Yes" ("T button name (\"OK\")")) -> (T button?=w265:bool)
        n149 = case shown="False" w265 {
          tunnel: ["Please Select your data folder" "Please Enter New Rig Name"] -> w264
          frame False {
            n150 = local write "Data Folder"(path "") -> ()
          }
          frame True {
          }
        }
      }
      frame "Please Enter New Rig Name" {
        n151 = global read "Preference_global.vi" "Rig Setup"() -> (w279:string)
        n152 = String Length(string=w279) -> (length=w284:i32)
        n153 = In Range and Coerce(upper limit=w281, x=w284, lower limit=w282) -> (In Range?=w280:bool)  [unwired: 1 out]
        n154 = case shown="False" w280 {
          tunnel: w279 -> [w291 w334]
          tunnel: [w287 "Update Rig setup menu ring"] -> w283
          tunnel: [w288 w334] -> w278
          tunnel: w282 -> [w290 _]
          tunnel: w281 -> [w289 _]
          frame False {
            n155 = stacked-sequence {
              seq-local: [w292 _] -> [_ w317]
              seq-local: [w299 _] -> [_ _]
              tunnel: w291 -> [w301 _]
              tunnel: w290 -> [w312 _]
              tunnel: w289 -> [w298 w315]
              tunnel: [_ w320] -> w288
              tunnel: [w304 _] -> w287
              frame #0 {
                n156 = Match Pattern(string=w301, regular expression="-") -> (before substring=w300:string, after substring=w299:string)  [unwired: 3 out]
                n157 = String Length(string=w299) -> (length=w297:i32)
                n158 = Subtract(x=w298, y=w297) -> (x-y=w296:i32)
                n159 = Format Into String(format string="Please Enter a Rig Name.\n It must be between %d and %d Characters" ("Message to user"), w312, w296) -> (resulting string=w311:string)  [unwired: 2 in, 1 out]
                n160 = call "Input_String_Dialog.vi"("Value"=w300, "Message to user"=w311) -> ("Ok Out"=w307:bool, "Output string"=w308:string)
                n161 = call "Fast_string_Replace.vi"("Replace match with:"="_", "Input String"=w308, "regular expression"=" ") -> ("Output String"=w293:string)  [unwired: 2 out]
                n162 = Select(t="Please Enter New Rig Name", s=w307, f="Save Preference File") -> (s? t:f=w304:string)
                n163 = call "Fast_string_Replace.vi"("Replace match with:"="_", "Input String"=w293, "regular expression"="-") -> ("Output String"=w292:string)  [unwired: 2 out]
              }
              frame #1 {
                n164 = String Length(string=w317) -> (length=w316:i32)
                n165 = Subtract(x=w315, y=w316) -> (x-y=w314:i32)
                n166 = Format Into String(format string="Please Enter a Rig Machine identifier if more than one machine per Rig.\n(Leave Blank for Rigs only using one Machine.)\nMust be less than %d Characters." ("Message to user"), w314) -> (resulting string=w313:string)  [unwired: 2 in, 1 out]
                n167 = call "Input_String_Dialog.vi"("Value"="", "Message to user"=w313) -> ("Output string"=w326:string)  [unwired: 1 out]
                n168 = call "Fast_string_Replace.vi"("Replace match with:"="_", "Input String"=w326, "regular expression"=" ") -> ("Output String"=w322:string)  [unwired: 2 out]
                n169 = call "Fast_string_Replace.vi"("Replace match with:"="_", "Input String"=w322, "regular expression"="-") -> ("Output String"=w319:string)  [unwired: 2 out]
                n170 = Empty String/Path?(string/path=w319) -> (empty?=w321:bool)
                n171 = case shown="False" w321 {
                  tunnel: [w329 w333] -> w320
                  tunnel: w317 -> [w332 w333]
                  tunnel: w319 -> [w330 _]
                  frame False {
                    n172 = Concatenate Strings(w332, "-" ("string"), w330) -> (w329:string)
                  }
                  frame True {
                  }
                }
              }
            }
          }
          frame True {
          }
        }
        n173 = global write "Preference_global.vi" "Rig Setup"(w278) -> ()
      }
      frame "Update Rig setup menu ring" {
        n174 = local read "Data Folder"() -> (w341:path)
        n175 = Build Path(base path=w341, name or relative path="Preferences") -> (appended path=w340:path)
        n176 = global read "Preference_global.vi" "Rig Setup"() -> (w347:string)
        n177 = Build Path(base path=w340, name or relative path=w338) -> (appended path=w339:path)
        n178 = List Folder(path=w339) -> (folder names=w337:string[])  [unwired: 1 in, 5 out]
        n179 = Build Array (concatenate)(w337, "--New Rig Setup--") -> (w343:string[])
        n180 = Search 1D Array(1D array=w343, element=w347) -> (index of element=w346:i32)  [unwired: 1 out]
        n181 = case shown="-1" w346 {
          tunnel: [w353 0] -> w349
          tunnel: w343 -> [w352 w356]
          tunnel: w347 -> [_ w355]
          tunnel: w346 -> [w353 _]
          tunnel: [w352 w354] -> w345
          frame 0, Default {
          }
          frame -1 {
            n182 = Build Array (concatenate)(w355, w356) -> (w354:string[])
          }
        }
        n183 = local write "Rig Setup"(w349) -> ()
        n184 = property on="Rig Setup" class="Ring (strict)"("Strings []"=w345) -> ()  [unwired: 2 in, 2 out]
      }
      frame "Update Constants Global" {
        n185 = global read "Preference_global.vi" "Rig Setup"() -> (w365:string)
        n186 = global read "Constants_global.vi" "Data Folder"() -> (w364:path)
        n187 = Build Path(base path=w364, name or relative path="Preferences") -> (appended path=w367:path)
        n188 = Build Path(base path=w367, name or relative path=w366) -> (appended path=w368:path)
        n189 = Build Path(base path=w368, name or relative path=w365) -> (appended path=w361:path)
        n190 = Build Path(base path=w361, name or relative path="ADAM table") -> (appended path=w373:path)
        n191 = Build Path(base path=w361, name or relative path="Serial") -> (appended path=w372:path)
        n192 = Build Path(base path=w361, name or relative path="All_Users") -> (appended path=w360:path)
        n193 = Build Path(base path=w367, name or relative path="Traverse_Setups") -> (appended path=w371:path)
        n194 = global write "Constants_global.vi" "ADAM setups folder"(w373) -> ()
        n195 = global write "Constants_global.vi" "Serial setups folder"(w372) -> ()
        n196 = global write "Constants_global.vi" "All_Users"(w360) -> ()
        n197 = global write "Constants_global.vi" "Traverse folder"(w371) -> ()
        n198 = Build Path(base path=w360, name or relative path="Collision_detection") -> (appended path=w358:path)
        n199 = global write "Constants_global.vi" "Collision_detection"(w358) -> ()
        n200 = Build Array(w373, w372, w360, w371) -> (w370:path[])
        n201 = for {
          tunnel: w370 -> [w382] mode=indexing
          n202 = Build Path(base path=w382, name or relative path="Test") -> (appended path=w380:path)
          n203 = call "Create_directory_path.vi"("Path name"=w380) -> ()  [unwired: 1 in, 2 out]
        }
      }
      frame "Post Processing Machine" {
        n204 = global read "Constants_global.vi" "Data Folder Local"() -> (w389:path)
        n205 = global read "Preference_global.vi" "User_Name"() -> (w384:string)
        n206 = Build Path(base path=w389, name or relative path="Preferences") -> (appended path=w391:path)
        n207 = Build Path(base path=w391, name or relative path=w384) -> (appended path=w385:path)
        n208 = Build Path(base path=w385, name or relative path="ADAM table") -> (appended path=w396:path)
        n209 = Build Path(base path=w385, name or relative path="Serial") -> (appended path=w395:path)
        n210 = Build Path(base path=w385, name or relative path="All_Users") -> (appended path=w386:path)
        n211 = Build Path(base path=w391, name or relative path="Traverse_Setups") -> (appended path=w394:path)
        n212 = local write "Post Processing Machine"(TRUE ("Post Processing Machine")) -> ()
        n213 = global write "Constants_global.vi" "ADAM setups folder"(w396) -> ()
        n214 = global write "Constants_global.vi" "Serial setups folder"(w395) -> ()
        n215 = global write "Constants_global.vi" "All_Users"(w386) -> ()
        n216 = global write "Constants_global.vi" "Traverse folder"(w394) -> ()
        n217 = Build Array(w396, w395, w386, w394) -> (w393:path[])
        n218 = for {
          tunnel: w393 -> [w405] mode=indexing
          n219 = Build Path(base path=w405, name or relative path="Test") -> (appended path=w403:path)
          n220 = call "Create_directory_path.vi"("Path name"=w403) -> ()  [unwired: 1 in, 2 out]
        }
        n221 = global write "Preference_global.vi" "Rig Setup"("Post_Processing_Machine" ("Rig Setup")) -> ()
      }
      frame "Copy Preferences?" {
        n222 = local read "Preferences for computer"() -> (w406:string)
        n223 = call "Setup_Filepath.vi"("Setup File Type"=Setup_Filetype."General", "Filename in"=w406) -> ("Filename Out"=w409:path)  [unwired: 1 out]
        n224 = call <vilib>:"Check if File or Folder Exists.vi"("path"=w409) -> ("file or folder exists?"=w408:bool)  [unwired: 1 in, 9 out]
        n225 = case shown="False" w408 {
          tunnel: w409 -> [w420 _]
          tunnel: [w418 TRUE ("file or folder exists?")] -> w407
          frame False {
            n226 = Strip Path(path=w420) -> (stripped path=w423:path)  [unwired: 1 out]
            n227 = Build Path(base path=w423, name or relative path="Preferences.xls") -> (appended path=w422:path)
            n228 = Move(source path=w422, 10:w420) -> (3:w419:path)  [unwired: 3 in, 2 out]
            n229 = call <vilib>:"Check if File or Folder Exists.vi"("path"=w419) -> ("file or folder exists?"=w418:bool)  [unwired: 1 in, 9 out]
          }
          frame True {
          }
        }
        n230 = case shown="False" w407 {
          tunnel: [w425 TRUE ("Error?")] -> w411
          frame False {
            n231 = global read "Constants_global.vi" "All_Users"() -> (w427:path)
            n232 = Build Path(base path=w427, name or relative path="Current_Username") -> (appended path=w428:path)
            n233 = call "Read_File_Simple.vi"("Filename"=w428) -> ("Error?"=w425:bool)  [unwired: 4 in, 5 out]
          }
          frame True {
          }
        }
        n234 = Select(t="Install Generic Meas Setup file", s=w411, f="Copy from last user") -> (s? t:f=w414:string)
      }
      frame "Copy from last user" {
        n235 = stacked-sequence {
          seq-local: [w447 _ _ _] -> [_ w457 w466 w478]
          seq-local: [_ w453 _ _] -> [_ _ _ w472]
          seq-local: [_ _ w461 _] -> [_ _ _ w471]
          tunnel: w434 -> [_ _ _ _]
          tunnel: [_ _ _ w470] -> w433
          frame #0 {
            n236 = global read "Constants_global.vi" "All_Users"() -> (w451:path)
            n237 = Seconds To Date/Time() -> (date time rec=w442:T12)  [unwired: 2 out]
            n238 = Unbundle By Name(w442) -> ("year"=w443:i32)
            n239 = global read "Preference_global.vi" "Rig Setup"() -> (w440:string)
            n240 = Build Path(base path=w451, name or relative path="Current_Username") -> (appended path=w449:path)
            n241 = Number To Decimal String(number=w443) -> (decimal integer string=w441:string)  [unwired: 1 out]
            n242 = global read "Constants_global.vi" "Data Folder"() -> (w446:path)
            n243 = call "Read_File_Simple.vi"("Filename"=w449) -> ("string"=w439:string)  [unwired: 4 in, 5 out]
            n244 = Build Path(base path=w446, name or relative path=w441) -> (appended path=w445:path)
            n245 = Build Path(base path=w445, name or relative path=w440) -> (appended path=w444:path)
            n246 = Build Path(base path=w444, name or relative path=w439) -> (appended path=w448:path)
            n247 = Build Path(base path=w448, name or relative path="Preferences") -> (appended path=w447:path)
          }
          frame #1 {
            n248 = local read "Preferences for computer"() -> (w452:string)
            n249 = call "Setup_Filepath.vi"("Setup File Type"=Setup_Filetype."General", "Filename in"=w452) -> ("Filename Out"=w455:path)  [unwired: 1 out]
            n250 = Build Path(base path=w457, name or relative path="General") -> (appended path=w459:path)
            n251 = Build Path(base path=w459, name or relative path=w452) -> (appended path=w458:path)
            n252 = Copy(10:w455, 11:w458) -> (0:w454:errorcluster)  [unwired: 3 in, 2 out]
            n253 = Unbundle By Name(w454) -> ("status"=w453:bool)
          }
          frame #2 {
            w464 = "Current_Setup.xls"
            n254 = Build Path(base path=w466, name or relative path="Meas Setups") -> (appended path=w468:path)
            n255 = Build Path(base path=w468, name or relative path=w464) -> (appended path=w467:path)
            n256 = call "Setup_Filepath.vi"("Setup File Type"=Setup_Filetype."Measurement Setups", "Filename in"=w464) -> ("Filename Out"=w463:path)  [unwired: 1 out]
            n257 = Copy(10:w463, 11:w467) -> (0:w462:errorcluster)  [unwired: 3 in, 2 out]
            n258 = Unbundle By Name(w462) -> ("status"=w461:bool)
          }
          frame #3 {
            w476 = "Current_Setup.xls"
            n259 = Build Path(base path=w478, name or relative path="Calib Setups") -> (appended path=w480:path)
            n260 = Build Path(base path=w480, name or relative path=w476) -> (appended path=w479:path)
            n261 = call "Setup_Filepath.vi"("Setup File Type"=Setup_Filetype."Calibration Setups", "Filename in"=w476) -> ("Filename Out"=w475:path)  [unwired: 1 out]
            n262 = Copy(10:w475, 11:w479) -> (0:w474:errorcluster)  [unwired: 3 in, 2 out]
            n263 = Unbundle By Name(w474) -> ("status"=w473:bool)
            n264 = Compound Arithmetic op=OR(w473, w472, w471) -> (w470:bool)
          }
        }
        n265 = Select(t="Install Generic Meas Setup file", s=w433, f="Read SW Preferences") -> (s? t:f=w431:string)
      }
      frame "Install Generic Meas Setup file" {
        n266 = global read "Constants_global.vi" "Run VI Folder"() -> (w492:path)
        n267 = Strip Path(path=w492) -> (stripped path=w490:path)  [unwired: 1 out]
        n268 = call "Setup_Filepath.vi"("Setup File Type"=Setup_Filetype."Measurement Setups", "Filename in"="Current_Setup.xls" ("name or relative path")) -> ("Filename Out"=w482:path)  [unwired: 1 out]
        n269 = Build Path(base path=w490, name or relative path="Templates") -> (appended path=w488:path)
        "Templates" <- w488
        n270 = call "Does_file_exist_(simple).vi"("Pathname"=w482) -> ("exists?"=w489:bool)
        n271 = case shown="False" w489 {
          tunnel: w482 -> [w498 _]
          tunnel: w488 -> [w496 _]
          frame False {
            n272 = Build Path(base path=w496, name or relative path="Measurement Setup.xls") -> (appended path=w495:path)
            n273 = Copy(10:w498, 11:w495) -> ()  [unwired: 1 in, 5 out]
          }
          frame True {
          }
        }
        n274 = Build Array (concatenate)(w485, w482) -> (w486:path[])
      }
      frame "Install Preference files" {
        n275 = local read "Preferences for computer"() -> (w499:string)
        n276 = Build Array(w499, w503, "Month_Names.xls" ("name or relative path"), "LDA_Configuration.xls") -> (w507:string[])
        n277 = for {
          tunnel: w507 -> [w511] mode=indexing
          tunnel: [w510] -> w501 mode=indexing
          n278 = call "Setup_Filepath.vi"("Setup File Type"=Setup_Filetype."General", "Filename in"=w511) -> ("Filename Out"=w510:path)  [unwired: 1 out]
          n279 = call "Does_file_exist_(simple).vi"("Pathname"=w510) -> ("exists?"=w513:bool)
          n280 = case shown="False" w513 {
            tunnel: w510 -> [w517 _]
            tunnel: w511 -> [w514 _]
            frame False {
              n281 = local read "Templates"() -> (w515:path)
              n282 = Build Path(base path=w515, name or relative path=w514) -> (appended path=w516:path)
              n283 = Copy(10:w517, 11:w516) -> ()  [unwired: 1 in, 5 out]
            }
            frame True {
            }
          }
        }
        n284 = Build Array (concatenate)(w502, w501) -> (w500:path[])
      }
      frame "Install Adam table files" {
        w522 = "Current_Setup.xls"
        n285 = global read "Constants_global.vi" "ADAM setups folder"() -> (w524:path)
        n286 = Build Path(base path=w524, name or relative path=w522) -> (appended path=w525:path)
        n287 = Build Path(base path=w524, name or relative path="Setup_Files") -> (appended path=w520:path)
        n288 = Build Array("Hi_Tec_Calibs.xls" ("name or relative path"), "A_Tunnel DB setup.xls" ("Substring"), "EnFlo_Tunnel DB setup.xls", "Aero_Tunnel DB setup.xls" ("name or relative path"), "D_Tunnel DB setup.xls") -> (w532:string[])
        n289 = Build Path(base path=w520, name or relative path=w522) -> (appended path=w519:path)
        n290 = for {
          tunnel: w532 -> [w536] mode=indexing
          tunnel: w524 -> [w537]
          n291 = Build Path(base path=w537, name or relative path=w536) -> (appended path=w535:path)
          n292 = call "Does_file_exist_(simple).vi"("Pathname"=w535) -> ("exists?"=w538:bool)
          n293 = case shown="False" w538 {
            tunnel: w535 -> [w542 _]
            tunnel: w536 -> [w539 _]
            frame False {
              n294 = local read "Templates"() -> (w540:path)
              n295 = Build Path(base path=w540, name or relative path=w539) -> (appended path=w541:path)
              n296 = Copy(10:w542, 11:w541) -> ()  [unwired: 1 in, 5 out]
            }
            frame True {
            }
          }
        }
        n297 = call "Create_directory_path.vi"("Path name"=w519) -> ("Path name Out"=w518:path)  [unwired: 1 in, 1 out]
        n298 = Move(source path=w525, 10:w518) -> ()  [unwired: 1 in, 5 out]
      }
      frame "Install Adam setup files" {
        w546 = "Current_Setup.xls"
        n299 = global read "Constants_global.vi" "ADAM setups folder"() -> (w548:path)
        n300 = Build Path(base path=w548, name or relative path="Setup_Files") -> (appended path=w545:path)
        n301 = Build Path(base path=w545, name or relative path=w546) -> (appended path=w543:path)
        n302 = call "Does_file_exist_(simple).vi"("Pathname"=w543) -> ("exists?"=w544:bool)
        n303 = case shown="False" w544 {
          tunnel: w543 -> [w559 _]
          tunnel: w546 -> [w557 _]
          frame False {
            n304 = local read "Templates"() -> (w558:path)
            n305 = Build Path(base path=w558, name or relative path="ADAM_Setup_files") -> (appended path=w556:path)
            n306 = Build Path(base path=w556, name or relative path=w557) -> (appended path=w555:path)
            n307 = Copy(10:w559, 11:w555) -> ()  [unwired: 1 in, 5 out]
          }
          frame True {
          }
        }
        n308 = Build Array (concatenate)(w550, w543) -> (w549:path[])
      }
      frame "Choose ADAM Setup file" {
        w568 = "Selected_Filename.txt" ("Substring")
        n309 = global read "Constants_global.vi" "ADAM setups folder"() -> (w572:path)
        n310 = Build Path(base path=w572, name or relative path="Setup_Files") -> (appended path=w569:path)
        n311 = Build Path(base path=w569, name or relative path=w568) -> (appended path=w567:path)
        n312 = call "Read_File_Simple.vi"("Filename"=w567) -> ("string"=w565:string)  [unwired: 2 in, 7 out]
        n313 = Build Array(w568) -> (w570:string[])
        n314 = call "List_files_in_order_of_age.vi"("Files to Hide"=w570, "Folder"=w569) -> ("file names"=w566:string[])
        n315 = Search 1D Array(1D array=w566, element=w565) -> (index of element=w562:i32)  [unwired: 1 out]
        n316 = property on="ADAM Setup File" class="Ring (strict)"("Strings []"=w566) -> ()  [unwired: 2 in, 2 out]
        n317 = Less Than 0?(x=w562) -> (x < 0?=w563:bool)
        n318 = Select(t=0, s=w563, f=w562) -> (s? t:f=w561:i32)
        n319 = local write "ADAM Setup File"(w561) -> ()
      }
      frame "Preference files continued" {
        n320 = Build Array("Hot_Wire_Bridges.txt", "Hot_Wire_Probes.txt", "Pressure_Transducers.txt") -> (w579:string[])
        n321 = for {
          tunnel: w579 -> [w587] mode=indexing
          tunnel: [w586] -> w577 mode=indexing
          n322 = call "Setup_Filepath.vi"("Setup File Type"=Setup_Filetype."Calibration Setups", "Filename in"=w587) -> ("Filename Out"=w586:path)  [unwired: 1 out]
          n323 = call "Does_file_exist_(simple).vi"("Pathname"=w586) -> ("exists?"=w589:bool)
          n324 = case shown="False" w589 {
            tunnel: w586 -> [w593 _]
            tunnel: w587 -> [w590 _]
            frame False {
              n325 = local read "Templates"() -> (w591:path)
              n326 = Build Path(base path=w591, name or relative path=w590) -> (appended path=w592:path)
              n327 = Copy(10:w593, 11:w592) -> ()  [unwired: 1 in, 5 out]
            }
            frame True {
            }
          }
        }
        n328 = Build Array (concatenate)(w578, w577) -> (w576:path[])
      }
      frame "Variable Names" {
        n329 = Build Array("Traverse to Traverse Collision Detection", "DataTranslation Device No.", "PWA Device Serial No.", "Analogue Device Serial No.", "Server address", "Server port number", "LabVIEW Administrators", "SMTP server IP address", "Server Comms", "Default Source Establishment Time (s)", "Temperature", "Abs Press (mbar)", "Default Traverse Name", "Tunnel Speed Control", "Current Overhead Factor", "EnFlo_Data_Central_Repository", "Auto Calib Error fr Previous", "Auto Calib Error fr First", "EnFlo_Data_Folder_Setup", "Use Triangle and Tree Collision Code", "Log Cameras if available", "Cameras to Log") -> (w616:string[])
        n330 = case shown="\"Load, Edit then Save\"" w610 {
          tunnel: ["Load From Preference file" w622 "Save Preference File"] -> w611
          frame "Load Preferences from file" {
          }
          frame "Load, Edit then Save" {
            n331 = local read "OK"() -> (w625:bool)
            n332 = Select(t="Save Preference File", s=w625, f="Load From Preference file") -> (s? t:f=w622:string)
          }
          frame "Save Preferences to file" {
          }
        }
      }
      frame "Load From Preference file" {
        n333 = local read "Preferences for computer"() -> (w627:string)
        n334 = call "Setup_Filepath.vi"("Setup File Type"=Setup_Filetype."General", "Filename in"=w627) -> ("Filename Out"=w628:path)  [unwired: 1 out]
        n335 = call "Read_File_Simple.vi"("Filename"=w628) -> ("string"=w636:string)  [unwired: 2 in, 7 out]
        n336 = for {
          tunnel: w638 -> [w641] mode=indexing
          tunnel: w636 -> [w640]
          w643 = FALSE  # Show Dialog?
          n337 = call "Get_Characters_from_string.vi"("Show Dialog?"=w643, "Input string"=w640, "Variable name"=w641) -> ("Status"=w642:enum16{"Char in string", "Char not in string"}, "Value"=w639:string)
          n338 = case shown="\"Char in string\"" w642 {
            tunnel: w641 -> [w645 _]
            tunnel: w639 -> [w644 _]
            frame "Char in string" {
              n339 = case shown="\"Cameras to Log\"" w645 {
                tunnel: w645 -> [w647 _ _ _ _ _ _ _ _ _ _ _ _ _ _ _ _ _ _ _ _ _ _]
                tunnel: w644 -> [_ w648 w649 w652 w653 w656 w657 w658 w660 w662 w665 w668 w671 w674 w676 _ w680 w684 w685 w687 w689 w692 w694]
                tunnel: w644 -> [_ _ _ _ _ _ _ _ _ _ _ _ _ _ _ w677 _ _ _ _ _ _ _]
                frame "No Match", Default {
                  n340 = call "Was_string_matched.vi"("Match Error"=TRUE, "Variable name"=w647) -> ()  [unwired: 1 in]
                }
                frame "Server address" {
                  n341 = global write "Preference_global.vi" "Server address"(w648) -> ()
                  n342 = local write "Server address"(w648) -> ()
                }
                frame "EnFlo_Data_Folder_Setup" {
                  n343 = local write "EnFlo_Data_Folder_Setup"(w649) -> ()
                  n344 = global write "Preference_global.vi" "EnFlo_Data_Folder_Setup"(w649) -> ()
                }
                frame "DataTranslation Device No." {
                  n345 = Decimal String To Number(string=w652, default (0L)=u32 0 ("default (0 I32)")) -> (number=w650:u32)  [unwired: 1 in, 1 out]
                  n346 = global write "Preference_global.vi" "DataTranslation Device No."(w650) -> ()
                  n347 = local write "DataTranslation Device No."(w650) -> ()
                }
                frame "Default Traverse Name" {
                  n348 = global write "Trav_pos_global.vi" "Default Traverse Setup"(w653) -> ()
                }
                frame "Server port number" {
                  n349 = Decimal String To Number(string=w656) -> (number=w655:i32)  [unwired: 3 out]
                  n350 = To Unsigned Long Integer(number=w655) -> (unsigned 32bit integer=w654:u32)
                  n351 = local write "Server port number"(w654) -> ()
                  n352 = global write "Preference_global.vi" "Server port number"(w654) -> ()
                }
                frame "Analogue Device Serial No." {
                  n353 = local write "Analogue Device Serial No."(w657) -> ()
                }
                frame "PWA Device Serial No." {
                  n354 = local write "PWA Device Serial No."(w658) -> ()
                }
                frame "Default Source Establishment Time (s)" {
                  n355 = Fract/Exp String To Number(string=w660) -> (number=w659:dbl)  [unwired: 4 out]
                  n356 = global write "Preference_global.vi" "Default Source Establishment Time (s)"(w659) -> ()
                  n357 = local write "Default Source Establishment Time (s)"(w659) -> ()
                }
                frame "Tunnel Speed Control" {
                  n358 = Equal?(x="TRUE", y=w662) -> (x = y?=w661:bool)
                  n359 = local write "Tunnel Speed Control"(w661) -> ()
                  n360 = global write "Preference_global.vi" "Tunnel Speed Control"(w661) -> ()
                }
                frame "Traverse to Traverse Collision Detection" {
                  n361 = Equal?(x="TRUE", y=w665) -> (x = y?=w664:bool)
                  n362 = global write "Preference_global.vi" "Traverse to Traverse Collision Detection"(w664) -> ()
                  n363 = local write "Traverse to Traverse Collision Detection"(w664) -> ()
                }
                frame "Log Cameras if available" {
                  n364 = Equal?(x="TRUE", y=w668) -> (x = y?=w667:bool)
                  n365 = global write "Preference_global.vi" "Log Cameras if available"(w667) -> ()
                  n366 = local write "Log Cameras if available"(w667) -> ()
                }
                frame "Use Triangle and Tree Collision Code" {
                  n367 = Equal?(x="TRUE", y=w671) -> (x = y?=w670:bool)
                  n368 = global write "Preference_global.vi" "Use New Collision Code"(w670) -> ()
                  n369 = local write "Use New Collision Code"(w670) -> ()
                }
                frame "LabVIEW Administrators" {
                  n370 = call "Get_array_values_fr_String.vi"("String Value"=w674) -> ("String array"=w673:string[])  [unwired: 1 out]
                  n371 = global write "Preference_global.vi" "LabVIEW Administrators"(w673) -> ()
                  n372 = local write "LabVIEW Administrators"(w673) -> ()
                }
                frame "Cameras to Log" {
                  n373 = call "Get_array_values_fr_String.vi"("String Value"=w676) -> ("String array"=w675:string[])  [unwired: 1 out]
                  n374 = global write "CamServer global.vi" "Demanded cameras"(w675) -> ()
                  n375 = local write "Cameras to Log"(w675) -> ()
                }
                frame "SMTP server IP address" {
                  n376 = local write "SMTP server IP address"(w677) -> ()
                  n377 = global write "Preference_global.vi" "SMTP server IP address"(w677) -> ()
                }
                frame "Server Comms" {
                  n378 = Equal?(x="TRUE", y=w680) -> (x = y?=w679:bool)
                  n379 = case shown="False" w679 {
                    tunnel: [Server_Comms."Do Not Link To Server" ("Server Comms") Server_Comms."Server Link Healthy" ("Server Comms")] -> w678
                    frame False {
                    }
                    frame True {
                    }
                  }
                  n380 = local write "Server Comms"(w678) -> ()
                  n381 = global write "Preference_global.vi" "Server Comms"(w678) -> ()
                }
                frame "Temperature" {
                  n382 = global write "Preference_global.vi" "Temperature"(w684) -> ()
                  n383 = local write "Temperature"(w684) -> ()
                }
                frame "Abs Press (mbar)" {
                  n384 = global write "Preference_global.vi" "Abs Press (mbar)"(w685) -> ()
                  n385 = local write "Abs Press (mbar)"(w685) -> ()
                }
                frame "EnFlo_Data_Central_Repository" {
                  n386 = String To Path(string=w687) -> (path=w686:path)
                  n387 = global write "Constants_global.vi" "EnFlo_Data_Central_Repository"(w686) -> ()
                }
                frame "Current Overhead Factor" {
                  n388 = Fract/Exp String To Number(string=w689) -> (number=w688:dbl)  [unwired: 4 out]
                  n389 = call "Overhead_Factor.vi"("Current Overhead Factor In"=w688, "Mode"=Overhead."Initialise totals to 3hr") -> ()  [unwired: 2 in, 1 out]
                }
                frame "Auto Calib Error fr Previous" {
                  n390 = Fract/Exp String To Number(string=w692) -> (number=w691:dbl)  [unwired: 4 out]
                  n391 = global write "Preference_global.vi" "% Error From Previous Calib"(w691) -> ()
                  n392 = local write "% Error From Previous Calib"(w691) -> ()
                }
                frame "Auto Calib Error fr First" {
                  n393 = Fract/Exp String To Number(string=w694) -> (number=w693:dbl)  [unwired: 4 out]
                  n394 = global write "Preference_global.vi" "% Error From First Calib"(w693) -> ()
                  n395 = local write "% Error From First Calib"(w693) -> ()
                }
              }
            }
            frame "Char not in string" {
            }
          }
        }
        n396 = local read "Post Processing Machine"() -> (w633:bool)
        n397 = Select(t="Check file permission status", s=w633, f="is traverse setup blank?") -> (s? t:f=w631:string)
        n398 = Build Array (concatenate)(w635, w628) -> (w634:path[])
      }
      frame "is traverse setup blank?" {
        n399 = local read "Data Folder"() -> (w701:path)
        n400 = global read "Trav_pos_global.vi" "Default Traverse Setup"() -> (w695:string)
        n401 = Build Path(base path=w701, name or relative path="Preferences") -> (appended path=w700:path)
        n402 = Build Path(base path=w700, name or relative path=w704) -> (appended path=w699:path)
        n403 = List Folder(path=w699) -> (folder names=w697:string[])  [unwired: 1 in, 5 out]
        n404 = Search 1D Array(1D array=w697, element=w695) -> (index of element=w698:i32)  [unwired: 1 out]
        n405 = case shown="0, Default" w698 {
          tunnel: w697 -> [_ w710]
          tunnel: [w708 w709] -> w696
          tunnel: w695 -> [w708 _]
          frame 0, Default {
          }
          frame -1 {
            n406 = Index Array(array=w710, index=0) -> (element=w709:string)
          }
        }
        n407 = global write "Trav_pos_global.vi" "Default Traverse Setup"(w696) -> ()
      }
      frame "Please Enter new  Traverse Setup" {
        n408 = global read "Trav_pos_global.vi" "Default Traverse Setup"() -> (w714:string)
        n409 = String Length(string=w714) -> (length=w719:i32)
        n410 = In Range and Coerce(upper limit=w716, x=w719, lower limit=w717) -> (In Range?=w715:bool)  [unwired: 1 out]
        n411 = case shown="False" w715 {
          tunnel: w714 -> [w730 w738]
          tunnel: ["Please Enter new  Traverse Setup" "Update Traverse setup menu ring"] -> w718
          tunnel: [w723 w738] -> w713
          tunnel: w717 -> [w727 _]
          tunnel: w716 -> [w726 _]
          frame False {
            n412 = Format Into String(format string="Please Enter a Traverse Setup Name\nIt must be between %d and %d Characters" ("Message to user"), w727, w726) -> (resulting string=w725:string)  [unwired: 2 in, 1 out]
            n413 = call "Input_String_Dialog.vi"("Value"=w730, "Message to user"=w725) -> ("Ok Out"=w722:bool, "Output string"=w724:string)
            n414 = case shown="False" w722 {
              tunnel: w724 -> [_ w735]
              tunnel: [w731 w734] -> w723
              frame False {
                n415 = property on="Default Traverse Name" class="Ring (strict)"() -> ("Strings []"=w732:string[])  [unwired: 2 in, 2 out]
                n416 = Index Array(array=w732, index=0) -> (element=w731:string)
              }
              frame True {
                n417 = call "Fast_string_Replace.vi"("Replace match with:"="_", "Input String"=w735, "regular expression"=" ") -> ("Output String"=w734:string)  [unwired: 2 out]
              }
            }
          }
          frame True {
          }
        }
        n418 = global write "Trav_pos_global.vi" "Default Traverse Setup"(w713) -> ()
      }
      frame "Update Traverse setup menu ring" {
        n419 = global read "Trav_pos_global.vi" "Default Traverse Setup"() -> (w743:string)
        n420 = local read "Data Folder"() -> (w749:path)
        n421 = Build Path(base path=w749, name or relative path="Preferences") -> (appended path=w748:path)
        n422 = Build Path(base path=w748, name or relative path=w741) -> (appended path=w747:path)
        n423 = List Folder(path=w747) -> (folder names=w745:string[])  [unwired: 1 in, 5 out]
        n424 = Build Array (concatenate)(w745, "--New Traverse Setup--") -> (w744:string[])
        n425 = Search 1D Array(1D array=w744, element=w743) -> (index of element=w751:i32)  [unwired: 1 out]
        n426 = case shown="-1" w751 {
          tunnel: [w757 0] -> w753
          tunnel: w744 -> [w756 w760]
          tunnel: w743 -> [_ w759]
          tunnel: w751 -> [w757 _]
          tunnel: [w756 w758] -> w742
          frame 0, Default {
          }
          frame -1 {
            n427 = Build Array (concatenate)(w759, w760) -> (w758:string[])
          }
        }
        n428 = local write "Default Traverse Name"(w753) -> ()
        n429 = property on="Default Traverse Name" class="Ring (strict)"("Strings []"=w742) -> ()  [unwired: 2 in, 2 out]
      }
      frame "Create Traverse setup" {
        n430 = local read "Templates"() -> (w763:path)
        n431 = Build Path(base path=w763, name or relative path="All_Traverses") -> (appended path=w769:path)
        n432 = stacked-sequence {
          seq-local: [w774 _] -> [_ w802]
          seq-local: [w773 _] -> [_ _]
          tunnel: w769 -> [w776 _]
          tunnel: [w779 _] -> w766
          tunnel: [w778 _] -> w765
          tunnel: w763 -> [_ w801]
          tunnel: [_ w799] -> w762
          frame #0 {
            w782 = "Default_Space_file.xls" ("name or relative path")
            w777 = "Traverse_Setup.xls" ("name or relative path")
            n433 = global read "Trav_pos_global.vi" "Default Traverse Setup"() -> (w773:string)
            n434 = global read "Constants_global.vi" "Traverse folder"() -> (w786:path)
            n435 = Build Path(base path=w776, name or relative path=w782) -> (appended path=w780:path)
            n436 = Build Path(base path=w776, name or relative path=w777) -> (appended path=w775:path)
            n437 = Build Path(base path=w786, name or relative path=w773) -> (appended path=w774:path)
            n438 = Build Path(base path=w774, name or relative path="Trav_Space_Files") -> (appended path=w783:path)
            n439 = Build Path(base path=w783, name or relative path=w782) -> (appended path=w779:path)
            n440 = call "Does_file_exist_(simple).vi"("Pathname"=w779) -> ("exists?"=w781:bool)
            n441 = case shown="False" w781 {
              tunnel: w780 -> [w789 _]
              tunnel: w779 -> [w788 _]
              frame False {
                n442 = call "Create_directory_path.vi"("Path name"=w788) -> ("Path name Out"=w787:path)  [unwired: 1 in, 1 out]
                n443 = Copy(10:w787, 11:w789) -> ()  [unwired: 1 in, 5 out]
              }
              frame True {
              }
            }
            n444 = Build Path(base path=w774, name or relative path=w777) -> (appended path=w778:path)
            n445 = call "Does_file_exist_(simple).vi"("Pathname"=w778) -> ("exists?"=w785:bool)
            n446 = case shown="False" w785 {
              tunnel: w775 -> [w798 _]
              tunnel: w778 -> [w794 _]
              tunnel: w773 -> [w797 _]
              frame False {
                w790 = TRUE  # append to file? (new file:F)
                n447 = call "Create_directory_path.vi"("Path name"=w794) -> ("Path name Out"=w793:path)  [unwired: 1 in, 1 out]
                n448 = call "Read_File_Simple.vi"("Filename"=w798) -> ("string"=w796:string)  [unwired: 2 in, 7 out]
                n449 = call "Fast_string_Replace.vi"("Replace match with:"=w797, "Input String"=w796, "regular expression"="A_Tunnel") -> ("Output String"=w792:string)  [unwired: 2 out]
                n450 = call "Write_Characters_To_File.vi"("file path (dialog if empty)"=w793, "advisory dialog? (display:T)"=TRUE, "character string"=w792, "append to file? (new file:F)"=w790) -> ()  [unwired: 1 in, 4 out]
              }
              frame True {
              }
            }
          }
          frame #1 {
            w800 = "Traverse_Preferences.txt" ("name or relative path")
            n451 = Build Path(base path=w802, name or relative path=w800) -> (appended path=w799:path)
            n452 = Build Path(base path=w801, name or relative path=w800) -> (appended path=w803:path)
            n453 = call "Does_file_exist_(simple).vi"("Pathname"=w799) -> ("exists?"=w804:bool)
            n454 = case shown="False" w804 {
              tunnel: w803 -> [w807 _]
              tunnel: w799 -> [w806 _]
              frame False {
                n455 = call "Create_directory_path.vi"("Path name"=w806) -> ("Path name Out"=w805:path)  [unwired: 1 in, 1 out]
                n456 = Copy(10:w805, 11:w807) -> ()  [unwired: 1 in, 5 out]
              }
              frame True {
              }
            }
          }
        }
        n457 = Build Array (concatenate)(w768, w765, w762, w766) -> (w767:path[])
      }
      frame "Check file permission status" {
        n458 = local read "Post Processing Machine"() -> (w808:bool)
        n459 = for {
          tunnel: w813 -> [w827] mode=indexing
          shift-right: [w824] -> w810
          shift-left: "" -> [w825]
          n460 = call "Can_File_be_Editted.vi"("Filename"=w827) -> ("File Permissions OK?"=w828:bool, "Comment String"=w826:string)  [unwired: 2 out]
          n461 = case shown="False" w828 {
            tunnel: w827 -> [w833 _]
            tunnel: w826 -> [w832 _]
            tunnel: w825 -> [w831 w834]
            tunnel: [w830 w834] -> w824
            frame False {
              n462 = Format Into String(format string="\"%s\" %s\n", initial string=w831, w833, w832) -> (resulting string=w830:string)  [unwired: 1 in, 1 out]
            }
            frame True {
            }
          }
        }
        n463 = case shown="\"Load, Edit then Save\"" w814 {
          tunnel: [w836 w840] -> w815
          tunnel: w808 -> [w835 w839]
          frame "Save Preferences to file", Default {
            n464 = Select(t="Save Preference File", s=w835, f="Output Dev Number") -> (s? t:f=w836:string)
          }
          frame "Load, Edit then Save" {
            n465 = Select(t="Data Folder Changed?", s=w839, f="What next1") -> (s? t:f=w840:string)
          }
        }
        n466 = Empty String/Path?(string/path=w810) -> (empty?=w811:bool)
        n467 = case shown="True" w811 {
          tunnel: w810 -> [w823 _]
          frame False {
            n468 = Concatenate Strings("The following file permissions need to be sorted out before the software will run correctly.\n\n" ("string"), w823) -> (w821:string)
            n469 = Two Button Dialog(message=w821, 1:"Continue" ("F button name (\"Cancel\")"), 2:"Abort" ("F button name (\"Cancel\")")) -> (T button?=w818:bool)
            n470 = Stop(stop? (T)=w818) -> ()
          }
          frame True {
          }
        }
      }
      frame "What next1" {
        n471 = property on="Rig Setup" class="Ring (strict)"() -> ("Strings []"=w845:string[])  [unwired: 2 in, 2 out]
        n472 = Array Size(array=w845) -> (size(s)=w849:i32)
        n473 = Decrement(x=w849) -> (x-1=w848:i32)
        n474 = Equal?(x=w848, y="Rig Setup") -> (x = y?=w847:bool)
        n475 = case shown="False" w847 {
          tunnel: [w853 "Please Enter New Rig Name" ("t")] -> w846
          tunnel: w845 -> [w856 _]
          tunnel: "Rig Setup" -> [w855 _]
          frame False {
            n476 = global read "Preference_global.vi" "Rig Setup"() -> (w857:string)
            n477 = Index Array(array=w856, index=w855) -> (element=w852:string)
            n478 = Not Equal?(x=w852, y=w857) -> (x != y?=w854:bool)
            n479 = case shown="False" w854 {
              tunnel: ["What next2" ("f") "Update Rig setup menu ring" ("t")] -> w853
              tunnel: w852 -> [_ w859]
              frame False {
              }
              frame True {
                n480 = global write "Preference_global.vi" "Rig Setup"(w859) -> ()
              }
            }
          }
          frame True {
            n481 = global write "Preference_global.vi" "Rig Setup"("") -> ()
          }
        }
      }
      frame "What next2" {
        n482 = property on="Default Traverse Name" class="Ring (strict)"() -> ("Strings []"=w865:string[])  [unwired: 2 in, 2 out]
        n483 = Array Size(array=w865) -> (size(s)=w869:i32)
        n484 = Decrement(x=w869) -> (x-1=w868:i32)
        n485 = Equal?(x=w868, y="Default Traverse Name") -> (x = y?=w867:bool)
        n486 = case shown="False" w867 {
          tunnel: [w873 "Please Enter new  Traverse Setup" ("t")] -> w866
          tunnel: w865 -> [w877 _]
          tunnel: "Default Traverse Name" -> [w876 _]
          frame False {
            n487 = global read "Trav_pos_global.vi" "Default Traverse Setup"() -> (w875:string)
            n488 = Index Array(array=w877, index=w876) -> (element=w872:string)
            n489 = Not Equal?(x=w872, y=w875) -> (x != y?=w874:bool)
            n490 = case shown="False" w874 {
              tunnel: ["Data Folder Changed?" ("f") "Update Traverse setup menu ring" ("t")] -> w873
              tunnel: w872 -> [_ w879]
              frame False {
              }
              frame True {
                n491 = global write "Trav_pos_global.vi" "Default Traverse Setup"(w879) -> ()
              }
            }
          }
          frame True {
            n492 = global write "Trav_pos_global.vi" "Default Traverse Setup"("") -> ()
          }
        }
      }
      frame "Data Folder Changed?" {
        w885 = "Please Select your data folder"
        n493 = global read "Constants_global.vi" "Data Folder"() -> (w891:path)
        n494 = local read "Data Folder"() -> (w892:path)
        n495 = property on="OK" class="Bool (strict)"("Visible"=TRUE) -> ()  [unwired: 2 in, 2 out]
        n496 = while {
          shift-right: [w901] -> _
          shift-left: _ -> [w900]
          tunnel: [w899] -> w887
          stop <- TRUE stop-if-true
          n497 = local read "Post Processing Machine"() -> (w901:bool)
          n498 = Not Equal?(x=w901, y=w900) -> (x != y?=w899:bool)
        }
        n499 = Not Equal?(x=w891, y=w892) -> (x != y?=w883:bool)
        n500 = Select(t=w885, s=w883, f="Has OK has been pressed?") -> (s? t:f=w884:string)
        n501 = case shown="True" w887 {
          tunnel: [w895 w897] -> w886
          tunnel: w885 -> [_ w897]
          tunnel: w884 -> [w895 _]
          frame False {
          }
          frame True {
            n502 = global write "Preference_global.vi" "Rig Setup"("") -> ()
          }
        }
      }
      frame "Has OK has been pressed?" {
        n503 = flat-sequence {
          tunnel: ["OK"] -> w903
          frame #0 {
            n504 = Wait (ms)(milliseconds to wait=u32 100) -> ()  [unwired: 1 out]
          }
          frame #1 {
          }
        }
        n505 = local read "Post Processing Machine"() -> (w904:bool)
        n506 = case shown="True" w903 {
          tunnel: w904 -> [w909 w915]
          tunnel: [w908 w912] -> w902
          frame False {
            n507 = Select(t="Data Folder Changed?", s=w909, f="What next1") -> (s? t:f=w908:string)
          }
          frame True {
            n508 = Select(t="Save Preference File", s=w915, f="Output Dev Number") -> (s? t:f=w912:string)
          }
        }
      }
      frame "Output Dev Number" {
        n509 = local read "Analogue Device Serial No."() -> (w923:string)
        n510 = local read "PWA Device Serial No."() -> (w924:string)
        n511 = for {
          tunnel: string[] ["Raw_Calibrations", "Raw_Measurements", "Results", "Calibrations", "Commands", "Pictures", "Videos"] -> [w931] mode=indexing
          tunnel: string[] ["Raw_Cal", "Raw_Meas", "Res", "Cal", "Cmd", "Pic", "Video"] -> [w929] mode=indexing
          n512 = call "Data_folder_Path.vi"("Data Type"=w931, "Short_Name"=w929) -> ("Data Folder"=w930:path)  [unwired: 4 in]
          n513 = Build Path(base path=w930, name or relative path="Test" ("Substring")) -> (appended path=w933:path)
          n514 = call "Create_directory_path.vi"("Path name"=w933) -> ()  [unwired: 1 in, 2 out]
        }
        n515 = global write "PWAtasksGLOBAL.vi" "PWA Dev Name"(w924) -> ()
        n516 = global write "PWAtasksGLOBAL.vi" "Analogue Dev Name"(w923) -> ()
        n517 = call "Data_folder_Path.vi"("Data Type"="Results_Post_Processed" ("element"), "Short_Name"="PP" ("ProjectNumberIn")) -> ("Data Folder"=w920:path)  [unwired: 4 in]
        n518 = call "Create_directory_path.vi"("Path name"=w920) -> ()  [unwired: 1 in, 2 out]
      }
      frame "Save Preference File" {
        n519 = call "Date_and_Time_to_string.vi"() -> ("Date and time (spreadsheet)"=w945:string)
        n520 = local read "Preferences for computer"() -> (w934:string)
        n521 = call "Setup_Filepath.vi"("Setup File Type"=Setup_Filetype."General", "Filename in"=w934) -> ("Filename Out"=w935:path)  [unwired: 1 out]
        n522 = for {
          tunnel: w944 -> [w955] mode=indexing
          shift-right: [w951] -> w943
          shift-left: w945 -> [w953]
          n523 = case shown="\"Cameras to Log\"" w955 {
            tunnel: w955 -> [w958 _ _ _ _ _ _ _ _ _ _ _ _ _ _ _ _ _ _ _ _ _ _]
            tunnel: ["No Match" "Server address" "EnFlo_Data_Folder_Setup" w962 w964 w966 w970 w974 w978 w982 w986 "SMTP server IP address" "PWA Device Serial No." "Analogue Device Serial No." w994 w995 w997 "Temperature" "Abs Press (mbar)" w1002 w1007 w1010 w1013] -> w954
            frame "No Match", Default {
              n524 = call "Was_string_matched.vi"("Match Error"=TRUE, "Variable name"=w958) -> ()  [unwired: 1 in]
            }
            frame "Server address" {
              n525 = global write "Preference_global.vi" "Server address"("Server address") -> ()
            }
            frame "EnFlo_Data_Folder_Setup" {
              n526 = global write "Preference_global.vi" "EnFlo_Data_Folder_Setup"("EnFlo_Data_Folder_Setup") -> ()
            }
            frame "Server port number" {
              n527 = global write "Preference_global.vi" "Server port number"("Server port number") -> ()
              n528 = Number To Decimal String(number="Server port number") -> (decimal integer string=w962:string)  [unwired: 1 out]
            }
            frame "Default Source Establishment Time (s)" {
              n529 = global write "Preference_global.vi" "Default Source Establishment Time (s)"("Default Source Establishment Time (s)") -> ()
              n530 = Number To Decimal String(number="Default Source Establishment Time (s)") -> (decimal integer string=w964:string)  [unwired: 1 out]
            }
            frame "Tunnel Speed Control" {
              n531 = global write "Preference_global.vi" "Tunnel Speed Control"("Tunnel Speed Control") -> ()
              n532 = Select(t="TRUE", s="Tunnel Speed Control", f="FALSE") -> (s? t:f=w966:string)
            }
            frame "Traverse to Traverse Collision Detection" {
              n533 = global write "Preference_global.vi" "Traverse to Traverse Collision Detection"("Traverse to Traverse Collision Detection") -> ()
              n534 = Select(t="TRUE", s="Traverse to Traverse Collision Detection", f="FALSE") -> (s? t:f=w970:string)
            }
            frame "Log Cameras if available" {
              n535 = global write "Preference_global.vi" "Log Cameras if available"("Log Cameras if available") -> ()
              n536 = Select(t="TRUE", s="Log Cameras if available", f="FALSE") -> (s? t:f=w974:string)
            }
            frame "Use Triangle and Tree Collision Code" {
              n537 = global write "Preference_global.vi" "Use New Collision Code"("Use New Collision Code") -> ()
              n538 = Select(t="TRUE", s="Use New Collision Code", f="FALSE") -> (s? t:f=w978:string)
            }
            frame "LabVIEW Administrators" {
              n539 = global write "Preference_global.vi" "LabVIEW Administrators"("LabVIEW Administrators") -> ()
              n540 = call "Put_Array_into_String.vi"("String array"="LabVIEW Administrators") -> ("String Value"=w982:string)
            }
            frame "Cameras to Log" {
              n541 = call "Analyse_string_array.vi"("String array"="Cameras to Log") -> ("Unique strings"=w984:string[])  [unwired: 1 in, 1 out]
              n542 = for {
                tunnel: w984 -> [w988] mode=indexing
                tunnel: [w988] -> w983 mode=indexing if=w987
                n543 = Not Equal?(x=w988, y="None") -> (x != y?=w987:bool)
              }
              n544 = call "Put_Array_into_String.vi"("String array"=w983) -> ("String Value"=w986:string)
              n545 = global write "CamServer global.vi" "Demanded cameras"(w983) -> ()
            }
            frame "SMTP server IP address" {
              n546 = global write "Preference_global.vi" "SMTP server IP address"("SMTP server IP address") -> ()
            }
            frame "PWA Device Serial No." {
            }
            frame "Analogue Device Serial No." {
            }
            frame "DataTranslation Device No." {
              n547 = global write "Preference_global.vi" "DataTranslation Device No."("DataTranslation Device No.") -> ()
              n548 = Number To Decimal String(number="DataTranslation Device No.") -> (decimal integer string=w994:string)  [unwired: 1 in]
            }
            frame "Default Traverse Name" {
              n549 = global read "Trav_pos_global.vi" "Default Traverse Setup"() -> (w995:string)
            }
            frame "Server Comms" {
              n550 = case shown="\"Server Link Healthy\"" "Server Comms" {
                tunnel: ["TRUE" "FALSE"] -> w997
                frame "Server Link Healthy" {
                }
                frame "Do Not Link To Server" {
                }
              }
              n551 = global write "Preference_global.vi" "Server Comms"("Server Comms") -> ()
            }
            frame "Temperature" {
              n552 = global write "Preference_global.vi" "Temperature"("Temperature") -> ()
            }
            frame "Abs Press (mbar)" {
              n553 = global write "Preference_global.vi" "Abs Press (mbar)"("Abs Press (mbar)") -> ()
            }
            frame "Current Overhead Factor" {
              n554 = call "Overhead_Factor.vi"("Mode"=Overhead."Read Current Overhead") -> ("Current Overhead Factor"=w1004:dbl)  [unwired: 3 in]
              n555 = Number To Fractional String(number=w1004, precision (6)=i16 4) -> (F-format string=w1002:string)  [unwired: 2 out]
            }
            frame "Auto Calib Error fr Previous" {
              n556 = global write "Preference_global.vi" "% Error From Previous Calib"("% Error From Previous Calib") -> ()
              n557 = Number To Fractional String(number="% Error From Previous Calib", precision (6)=i16 2) -> (F-format string=w1007:string)  [unwired: 2 out]
            }
            frame "Auto Calib Error fr First" {
              n558 = global write "Preference_global.vi" "% Error From First Calib"("% Error From First Calib") -> ()
              n559 = Number To Fractional String(number="% Error From First Calib", precision (6)=i16 2) -> (F-format string=w1010:string)  [unwired: 2 out]
            }
            frame "EnFlo_Data_Central_Repository" {
              n560 = global read "Constants_global.vi" "EnFlo_Data_Central_Repository"() -> (w1012:path)
              n561 = Path To String(path=w1012) -> (string=w1013:string)
            }
          }
          n562 = call "Characters_to_string.vi"("Characters to write"=w954, "Label for characters"=w955) -> ("Output string"=w952:string)
          n563 = Concatenate Strings(w953, w952) -> (w951:string)
        }
        n564 = case shown="\"Load, Edit then Save\"" w939 {
          tunnel: [TRUE TRUE TRUE] -> w938
          frame "Load, Edit then Save" {
            n565 = Current VI's Path() -> (path=w947:path)
            n566 = call "Open_Close_Front_Panel.ph.vi"("Front Panel Window:Open"=FALSE, "VI path"=w947) -> ()  [unwired: 2 out]
          }
          frame "Load Preferences from file" {
          }
          frame "Save Preferences to file" {
          }
        }
        n567 = call "Write_Characters_To_File.vi"("file path (dialog if empty)"=w935, "advisory dialog? (display:T)"=FALSE, "character string"=w943, "append to file? (new file:F)"=FALSE) -> ()  [unwired: 1 in, 4 out]
      }
      frame "Save SW Preferences" {
        w1033 = FALSE  # append to file? (new file:F)
        w1034 = FALSE  # advisory dialog? (display:T)
        n568 = local read "Post Processing Machine"() -> (w1023:bool)
        n569 = global read "Preference_global.vi" "User_Name"() -> (w1016:string)
        n570 = Path To String(path="Data Folder") -> (string=w1025:string)
        n571 = global read "Preference_global.vi" "Server Comms"() -> (w1029:T4)
        n572 = call "Characters_to_string.vi"("Characters to write"=w1025, "Label for characters"=w1027) -> ("Output string"=w1035:string)
        n573 = Select(t="True", s=w1023, f="False") -> (s? t:f=w1020:string)
        n574 = call "Characters_to_string.vi"("Characters to write"=w1016, "Label for characters"=w1017) -> ("Output string"=w1015:string)
        n575 = call "Characters_to_string.vi"("Characters to write"=w1020, "Label for characters"=w1018) -> ("Output string"=w1019:string)
        n576 = call "Date_and_Time_to_string.vi"() -> ("Date and time (spreadsheet)"=w1030:string)
        n577 = case shown="\"Server Link Healthy\"" w1029 {
          tunnel: ["Update Served VI file" "Update Local Adam Table"] -> w1028
          frame "Server Link Healthy" {
          }
          frame "Do Not Link To Server" {
          }
        }
        n578 = Concatenate Strings(w1030, w1035, w1019, w1015) -> (w1031:string)
        n579 = local read "EnFlo SW Preferences"() -> (w1032:path)
        n580 = call "Write_Characters_To_File.vi"("file path (dialog if empty)"=w1032, "advisory dialog? (display:T)"=w1034, "character string"=w1031, "append to file? (new file:F)"=w1033) -> ()  [unwired: 1 in, 4 out]
        n581 = case shown="True" "Reset Email Counter" {
          tunnel: "Reset Email Counter" -> [_ w1038]
          frame False {
          }
          frame True {
            n582 = global write "Preference_global.vi" "Unblock Email"(w1038) -> ()
          }
        }
      }
      frame "Update Local Adam Table" {
        n583 = stacked-sequence {
          seq-local: [w1050 _] -> [_ w1064]
          tunnel: ["Update Served VI file" _] -> w1042
          frame #0 {
            w1050 = T13 {"Ch Name"="", "Type"="", "Function"=enum."Analogue Input", "Ch State"=enum."On", "Calibration type"=enum."Raw", "A"=0.0, "B"=0.0, "C"=0.0, "D"=0.0, "Comments"="", "Address"={"Main"=0, "Ch."=0, "Sub"=0, "Port Name"=""}, "String"="", "Duty"=0} ("Ch Discription")
            n584 = global read "Preference_global.vi" "Abs Press (mbar)"() -> (w1047:string)
            n585 = global read "Preference_global.vi" "Temperature"() -> (w1048:string)
            n586 = Bundle By Name(cluster=w1050, "Type"=T10 "", "Calibration type"=Calib_type_ADAM."Raw", "A"=1.0) -> (w1051:T13)
            n587 = Build Array(w1048, w1047) -> (w1046:string[])
            n588 = for {
              tunnel: [w1057] -> w1049 mode=indexing
              tunnel: w1051 -> [w1056]
              tunnel: w1046 -> [w1055] mode=indexing
              n589 = Bundle By Name(cluster=w1056, "Ch Name"=w1055) -> (w1057:T13)
            }
            n590 = call "Update_Ch_Discription_client.vi"("Channels to update In"=w1049) -> ()  [unwired: 1 out]
          }
          frame #1 {
            n591 = global read "Preference_global.vi" "Rig Setup"() -> (w1059:string)
            n592 = call "Get_Current_Scan_client.vi"() -> ("Ch Description Array"=w1065:T13[])  [unwired: 1 in, 3 out]
            n593 = Match Pattern(string=w1059, regular expression="-") -> (before substring=w1058:string)  [unwired: 4 out]
            n594 = Format Into String(format string="%s Metadata:" ("Format String"), w1058) -> (resulting string=w1067:string)  [unwired: 2 in, 1 out]
            n595 = Initialize Array(w1064, 0 ("dimension size")) -> (w1062:T13[])
            n596 = for {
              shift-right: [w1078] -> w1061
              shift-left: w1062 -> [w1079]
              tunnel: w1065 -> [w1070] mode=indexing
              tunnel: w1067 -> [w1077]
              tunnel: "Metadata:" ("Format String") -> [w1076]
              n597 = Unbundle By Name(w1070) -> ("Ch Name"=w1069:string)
              n598 = Match Pattern(string=w1069, regular expression=w1077) -> (offset past match=w1074:i32)  [unwired: 4 out]
              n599 = Match Pattern(string=w1069, regular expression=w1076) -> (offset past match=w1075:i32)  [unwired: 4 out]
              n600 = Greater Or Equal To 0?(x=w1075) -> (x >= 0?=w1072:bool)
              n601 = Less Than 0?(x=w1074) -> (x < 0?=w1073:bool)
              n602 = And(x=w1073, y=w1072) -> (x .and. y?=w1071:bool)
              n603 = case shown="True" w1071 {
                tunnel: w1079 -> [w1080 w1085]
                tunnel: [w1080 w1084] -> w1078
                tunnel: w1070 -> [_ w1083]
                frame False {
                }
                frame True {
                  n604 = Bundle By Name(cluster=w1083, "Ch State"=Channel_State."Off") -> (w1081:T13)
                  n605 = Build Array (concatenate)(w1085, w1081) -> (w1084:T13[])
                }
              }
            }
            n606 = call "Update_Ch_Discription_client.vi"("Channels to update In"=w1061) -> ()  [unwired: 1 out]
          }
        }
      }
      frame "Update Served VI file" {
        # "Template"
        # "Orig"
        n607 = call "Setup_Filepath.vi"("Setup File Type"=Setup_Filetype."General", "Filename in"=w1087) -> ("Filename Out"=w1086:path)  [unwired: 1 out]
        n608 = Build Array("Served:VI:Name", "Served:VI:Path", "Server:IP Number:& Port No") -> (w1092:string[])
        n609 = stacked-sequence {
          seq-local: [w1097 _ _ _] -> [_ _ w1107 _]
          seq-local: [_ w1104 _ _] -> [_ _ w1108 _]
          seq-local: [_ _ w1109 _] -> [_ _ _ w1133]
          tunnel: w1092 -> [w1099 w1105 _ w1134]
          tunnel: w1086 -> [w1098 _ _ w1135]
          tunnel: w1087 -> [_ w1101 _ _]
          frame #0 {
            n610 = call "Read_Ch_data_file.vi"("Present Channels"=w1099, "Output"=enum16{"All Ch data", "The last few rows"}."All Ch data", "Filename"=w1098) -> ("Channel Values"=w1097:string[][])  [unwired: 2 in, 4 out]
          }
          frame #1 {
            n611 = local read "Templates"() -> (w1103:path)
            n612 = Build Path(base path=w1103, name or relative path=w1101) -> (appended path=w1102:path)
            n613 = call "Read_Ch_data_file.vi"("Present Channels"=w1105, "Output"=enum16{"All Ch data", "The last few rows"}."All Ch data", "Filename"=w1102) -> ("Channel Values"=w1104:string[][])  [unwired: 2 in, 4 out]
          }
          frame #2 {
            n614 = Index Array(array=w1107, index (col)=0 ("Index")) -> (element=w1112:string[])  [unwired: 1 in]
            n615 = To Upper Case(1:w1108) -> (0:w1110:string[][])
            n616 = To Upper Case(1:w1112) -> (0:w1111:string[])
            n617 = for {
              tunnel: w1111 -> [w1115]
              tunnel: w1108 -> [w1120] mode=indexing
              tunnel: w1110 -> [w1114] mode=indexing
              tunnel: [w1117] -> w1109 mode=indexing
              tunnel: w1107 -> [w1116]
              n618 = Index Array(array=w1114, index=0 ("Index")) -> (element=w1118:string)
              n619 = Search 1D Array(1D array=w1115, element=w1118) -> (index of element=w1119:i32)  [unwired: 1 out]
              n620 = case shown="0, Default" w1119 {
                tunnel: w1120 -> [w1129 w1130]
                tunnel: w1119 -> [w1126 _]
                tunnel: [w1122 w1130] -> w1117
                tunnel: w1116 -> [w1127 _]
                frame 0, Default {
                  n621 = Index Array(array=w1127, index (row)=w1126, index (col)=2 ("Index")) -> (element=w1124:string)
                  n622 = Array Subset(array=w1129, length=2) -> (w1123:string[])  [unwired: 1 in]
                  n623 = Build Array (concatenate)(w1123, w1124) -> (w1122:string[])
                }
                frame -1 {
                }
              }
            }
          }
          frame #3 {
            w1131 = FALSE  # Append last row only
            w1132 = FALSE  # exists?
            n624 = call "Write_Ch_data_file.vi"("Append last row only"=w1131, "exists?"=w1132, "Channel Values"=w1133, "Channel names"=w1134, "Filename"=w1135) -> ()  [unwired: 3 in, 4 out]
          }
        }
      }
      frame "Initialise Globals" {
        w1140 = TRUE  # OK
        w1144 = FALSE  # append to file? (new file:F)
        w1143 = FALSE  # advisory dialog? (display:T)
        n625 = global read "Constants_global.vi" "ADAM setups folder"() -> (w1150:path)
        n626 = global read "Constants_global.vi" "All_Users"() -> (w1139:path)
        n627 = property on="ADAM Setup File" class="Ring (strict)"() -> ("Strings []"=w1145:string[])  [unwired: 2 in, 2 out]
        n628 = Build Path(base path=w1139, name or relative path="Current_Username") -> (appended path=w1137:path)
        n629 = Build Path(base path=w1150, name or relative path="Setup_Files") -> (appended path=w1148:path)
        n630 = global read "Preference_global.vi" "User_Name"() -> (w1136:string)
        n631 = Build Path(base path=w1148, name or relative path="Selected_Filename.txt" ("Substring")) -> (appended path=w1141:path)
        n632 = call "Get_users_email_addresses.vi"("OK"=w1140) -> ()  [unwired: 5 out]
        n633 = Index Array(array=w1145, index="ADAM Setup File") -> (element=w1142:string)
        n634 = call "Write_File_Simple.vi"("character string"=w1136, "file path"=w1137) -> ()  [unwired: 1 in, 2 out]
        n635 = call "Write_Characters_To_File.vi"("file path (dialog if empty)"=w1141, "advisory dialog? (display:T)"=w1143, "character string"=w1142, "append to file? (new file:F)"=w1144) -> ()  [unwired: 1 in, 4 out]
      }
    }
  }
